vi "Automatic_IV_CV_with_XML_Global_Stop_V1.1.vi"() -> ()   [LabVIEW 2009]
uses:
  subVIs/CMSFPIX_LV80.llb/Keith 237 Operate/Standby.vi
  <vilib>/xml/Close Reference(Node).vi
  <vilib>/Utility/file.llb/Write To Spreadsheet File (string).vi
  <vilib>/Utility/file.llb/Write To Spreadsheet File (DBL).vi
  <vilib>/xml/NI_XML.lvlib
panel:
  in  "File Path":path=path "C:/Documents and Settings/PROBER/Desktop/Andrew_Test/VI Test Output"
  out "voltage \ncompliance level":dbl=1e-05
  out "Wafer Number":string
  out "Contact Check Result":string="Skipped"
  out "Site Number":i32
  out "File Name":string
  in  "Tab Control 2":enum32{"IV Check", "CV Check"}(tab)
  out "Boolean":bool caption="Voltage Breakdown"
  out "Boolean 2":bool caption="Leakage Current Check Total"
  out "Boolean 3":bool caption="Leakage Current Check Active"
  out "Boolean 4":bool caption="Leakage Current Check Guardring"
  out "Boolean 5":bool caption="150V Bias Check"
  out "Contact Check":bool
  out "Status":string
  out "Bias Polarity":dbl=1.0 format="%.2f"
  out "1/C^2":cluster{"Y":dbl[], "Y":dbl[]}[](graph)
  out "semaphore":T1
  out "voltage \ncompliance cutoff":dbl=1e-05
  in  "Tab Control":enum32{"Site Selection"}(tab)
  in  "Site 1":bool=TRUE
  in  "Site 2":bool=TRUE
  in  "Site 3":bool=TRUE
  in  "Site 4":bool=TRUE
  in  "Site 5":bool=TRUE
  in  "Site 6":bool=TRUE
  in  "Site 7":bool=TRUE
  in  "Site 8":bool=TRUE
  in  "Site 9":bool=TRUE
  in  "Site 10":bool=TRUE
  in  "Site 11":bool=TRUE
  in  "Site 12":bool=TRUE
  in  "Site 13":bool=TRUE
  in  "Site 14":bool=TRUE
  in  "Site 15":bool=TRUE
  in  "Site 16":bool=TRUE
  in  "Site 17":bool=TRUE
  in  "Site 18":bool=TRUE
  in  "Site 19":bool=TRUE
  in  "Site 20":bool=TRUE
  in  "Site 21":bool=TRUE
  in  "Site 22":bool=TRUE
  in  "Running Conditional":bool
  out "error out 7":T2
  in  "IV or CV":i32
  in  "Emergency Stop":bool
  out "error out 6":T2
  in  "Stop Loop":bool=TRUE
  in  "Total Site # CV":i32=12
  out "Secondary Parameter":u16(ring) items=["None", "Cs", "Cp", "Ls", "Lp", "Rs", "Rp", "DF", "Q", "Z", "Y", "Phase", "ESR", "Gp", "Xs", "Bp"]
  out "Auto Compliance":dbl=9.9e-05
  out "Compliance":dbl=1e-09
  out "Compliance":bool
  out "Total Current":dbl format="%#_6e"
  out "Secondary Parameter Graph":cluster{"Y":dbl[], "Y":dbl[]}[](graph) caption="DF"
  in  "Absolute?":bool
  out "Voltage Range":string
  out "Primary Parameter":u16(ring)=2 items=["AUTO", "Cs", "Cp", "Ls", "Lp", "Rs", "Rp", "DF", "Q", "Z", "Y", "Phase", "ESR", "Gp", "Xs", "Bp"]
  out "Time Delay mS":dbl=20.0
  out "Number of Averages":dbl=1.0
  out "Voltage Level":dbl=1.0
  out "Frequency":dbl=1000.0
  in  "Bias Loop":bool
  out "K237_Bias":dbl
  in  "Archive":T3(tab)=enum."Primary"
  out "Diode Total Current Archive":cluster{"Y":dbl[], "Y":dbl[]}[](graph) caption="Total Current"
  out "Diode GRD Archive":cluster{"Y":dbl[], "Y":dbl[]}[](graph)
  out "Diode ACTIVE Archive":cluster{"Y":dbl[], "Y":dbl[]}[](graph)
  out "Single Chip Total Current Archive":cluster{"Y":dbl[], "Y":dbl[]}[](graph) caption="Total Current"
  out "Single Chip GRD Archive":cluster{"Y":dbl[], "Y":dbl[]}[](graph)
  out "Single Chip ACTIVE Archive":cluster{"Y":dbl[], "Y":dbl[]}[](graph)
  out "2x8 Total Current Archive":cluster{"Y":dbl[], "Y":dbl[]}[](graph) caption="Total Current"
  out "2x8 GRD Archive":cluster{"Y":dbl[], "Y":dbl[]}[](graph)
  out "2x8 ACTIVE Archive":cluster{"Y":dbl[], "Y":dbl[]}[](graph)
  out "Slim-Edge ACTIVE Archive":cluster{"Y":dbl[], "Y":dbl[]}[](graph)
  out "Slim-Edge GRD Archive":cluster{"Y":dbl[], "Y":dbl[]}[](graph)
  out "Slim-Edge Total Current Archive":cluster{"Y":dbl[], "Y":dbl[]}[](graph) caption="Total Current"
  out "Single Chip Capacitance":cluster{"Y":dbl[], "Y":dbl[]}[](graph)
  out "2x8 Chip Capacitance":cluster{"Y":dbl[], "Y":dbl[]}[](graph)
  out "Diodes Capacitance":cluster{"Y":dbl[], "Y":dbl[]}[](graph)
  in  "Halt CV":bool
  in  "Halt IV":bool
  out "Running?":bool
  in  "Total Site # IV":i32=22
  out "Site # CV":dbl
  out "Site # IV":dbl
  out "error out":errorcluster
  in  "CV-V-Limit":i32=10
  out "Capacitance":cluster{"Y":dbl[], "Y":dbl[]}[](graph) caption="Cp"
  in  "CV-V-Steps":i32=1
  out "QuadTech Status":string
  out "Total Current":cluster{"Y":dbl[], "Y":dbl[]}[](graph)
  out "6485 GRD (GPIB 10)":cluster{"Y":dbl[], "Y":dbl[]}[](graph)
  out "6485 ACTIVE (GPIB 14)":cluster{"Y":dbl[], "Y":dbl[]}[](graph)
  out "error out 5":errorcluster
  out "error out 4":errorcluster
  in  "IV-V-Steps":i32=1
  in  "IV-V-Limit":i32=10
  in  "error in (no error)":errorcluster
  # "Note: The Total Site # indexes\nstarting at 0 and goes to n-1,\nso if there are a total of 3 sites\nthen Total Site # should be set\nto 3"
  # "Note 2: This code is setup for a specific\nwafer map. If a map with a different\nnumber of subsites and/or different layout\nis used the naming will be incorrect"
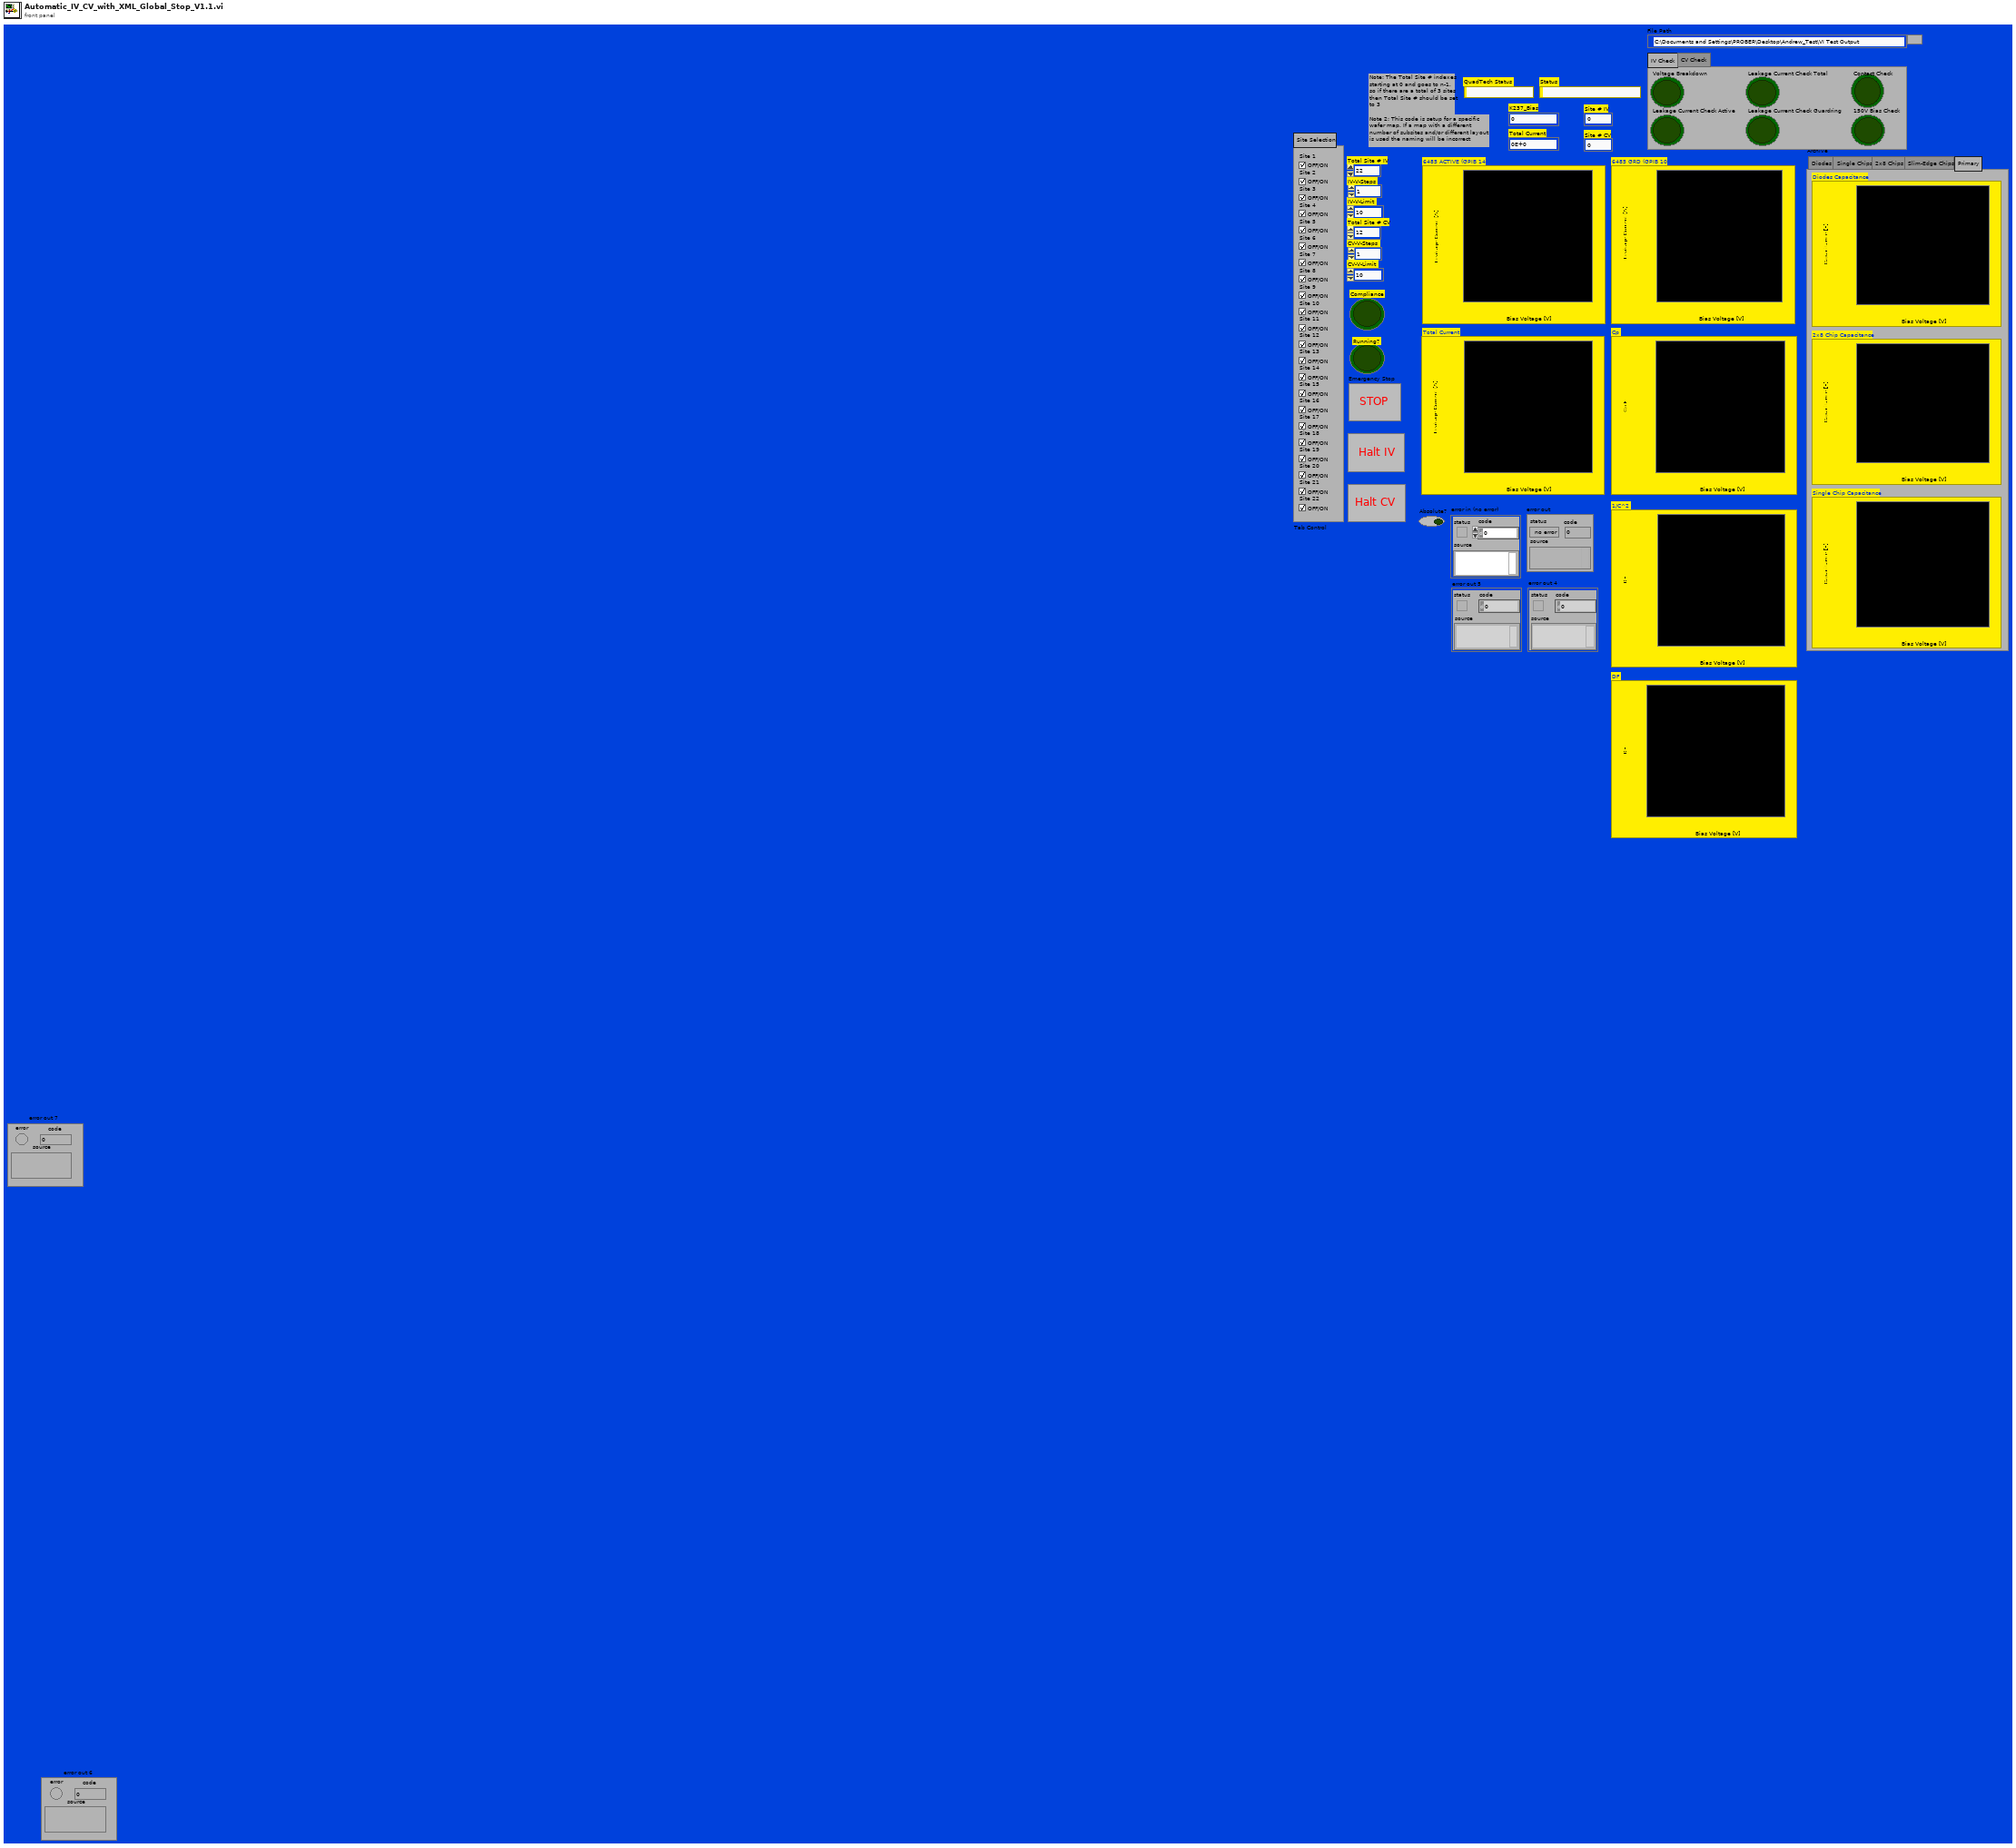
[diagram p1: front panel]
types:
  T1 = typedef "Semaphore RefNum" = refnum<k1>
  T2 = cluster{"error":bool, "code":i32, "source":string}
  T3 = enum32{"Diodes", "Single Chips", "2x8 Chips", "Slim-Edge Chips", "Primary"}
  T4 = cluster{"Name of Test":string, string, "Comment Description":string, "User":string}
  T5 = enum16{"open", "replace", "create", "open or create", "replace or create", "replace or create with confirmation"}
  T6 = cluster{cluster{"Y":dbl[], "Y":dbl[]}[], cluster{"Y":dbl[], "Y":dbl[]}[], cluster{"Y":dbl[], "Y":dbl[]}[], cluster{"Y":dbl[], "Y":dbl[]}[], cluster{"Y":dbl[], "Y":dbl[]}[], cluster{"Y":dbl[], "Y":dbl[]}[], cluster{"Y":dbl[], "Y":dbl[]}[], cluster{"Y":dbl[], "Y":dbl[]}[], cluster{"Y":dbl[], "Y":dbl[]}[], cluster{"Y":dbl[], "Y":dbl[]}[], cluster{"Y":dbl[], "Y":dbl[]}[], cluster{"Y":dbl[], "Y":dbl[]}[]}
  T7 = enum16{"Left Button", "Center Button", "Right Button", "Window Close"}
  T8 = cluster{"error":bool, "code":i8, "source":string}
  T9 = cluster{cluster{"Y":dbl[], "Y":dbl[]}[], cluster{"Y":dbl[], "Y":dbl[]}[], cluster{"Y":dbl[], "Y":dbl[]}[]}
  T10 = cluster{"Primary ":string, "Primary Value":string, "Primary Unit":string, "Secondary":string, "Secondary Value":string, "Secondary Unit":string}
  T11 = cluster{"XY Graph":cluster{"Y":dbl[], "Y":dbl[]}[], "XY Graph":cluster{"Y":dbl[], "Y":dbl[]}[], "XY Graph":cluster{"Y":dbl[], "Y":dbl[]}[]}
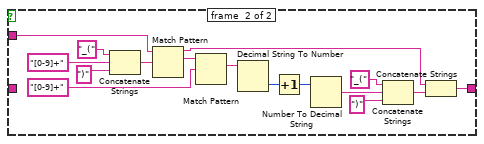
[diagram p2: hidden frame]
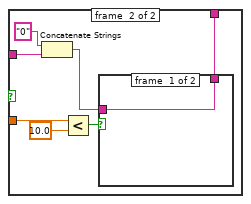
[diagram p4: hidden frame]
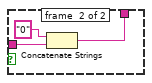
[diagram p5: hidden frame]
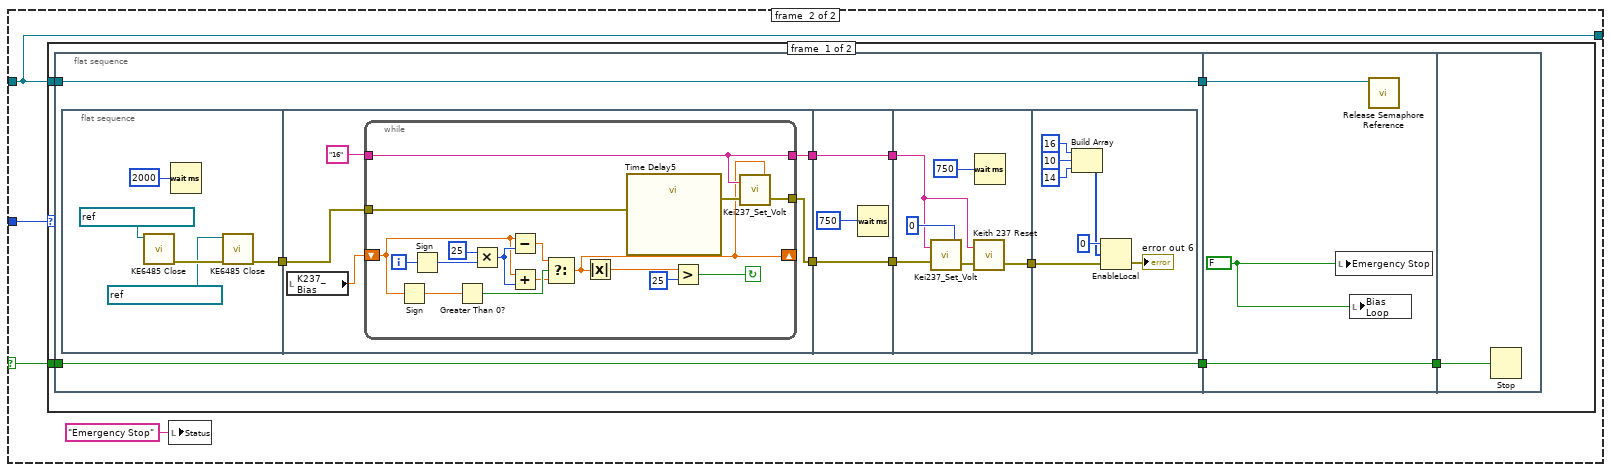
[diagram p7: hidden frame]
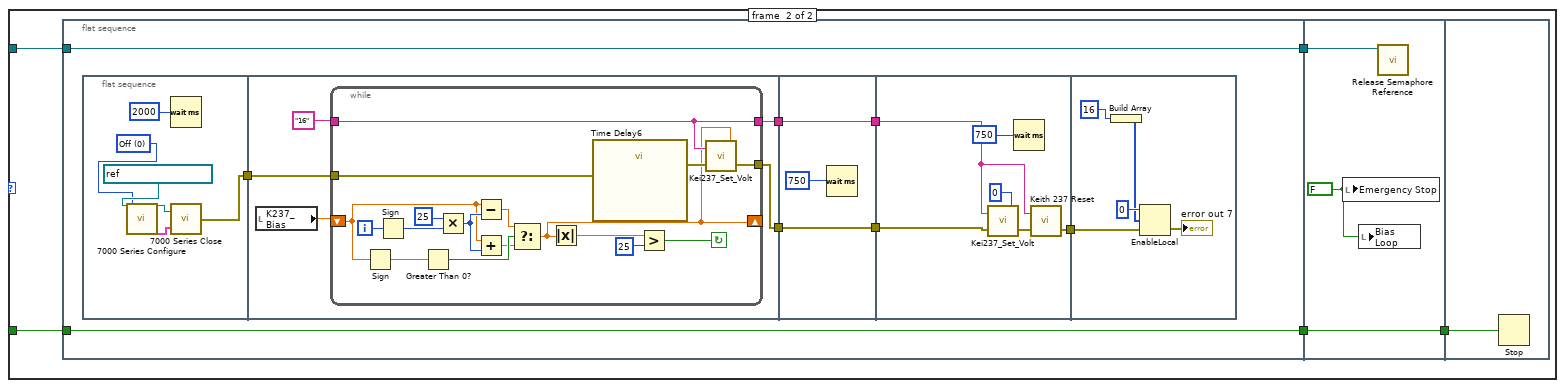
[diagram p8: hidden frame]
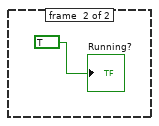
[diagram p9: hidden frame]
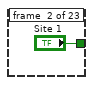
[diagram p10: hidden frame]
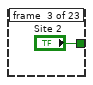
[diagram p11: hidden frame]
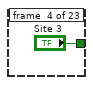
[diagram p12: hidden frame]
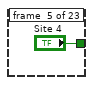
[diagram p13: hidden frame]
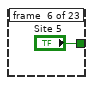
[diagram p14: hidden frame]
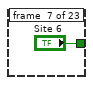
[diagram p15: hidden frame]
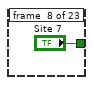
[diagram p16: hidden frame]
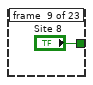
[diagram p17: hidden frame]
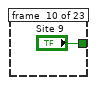
[diagram p18: hidden frame]
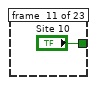
[diagram p19: hidden frame]
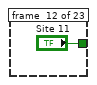
[diagram p20: hidden frame]
diagram:
  (unwired) path "" ("base path")
  # "Wafer Folder"
  # "Test Name Subfolder"
  # "XML Subfolder"
  # "Single Chip"
  # "2x8"
  # "Diode"
  # "Total"
  # "GRD"
  # "Active"
  # "Capacitance"
  # "Slim-Edge"
  # "2x8"
  # "Single Chip"
  # "Diodes"
  # "Change wiring to CV"
  # "DO CV MEASUREMENTS"
  # "Do CV measurements"
  # "Configure CV instuments"
  # "Do IV measurements"
  # "Configure IV instuments"
  # "DO IV MEASUREMENTS"
  n1 = invoke on="Diode ACTIVE Archive" class="XYGraph (strict)" method="Reinit To Default"() -> ()  [unwired: 3 in, 3 out]
  n2 = invoke on="Diode GRD Archive" class="XYGraph (strict)" method="Reinit To Default"() -> ()  [unwired: 3 in, 3 out]
  n3 = invoke on="Diode Total Current Archive" class="XYGraph (strict)" method="Reinit To Default"() -> ()  [unwired: 3 in, 3 out]
  n4 = invoke on="Diodes Capacitance" class="XYGraph (strict)" method="Reinit To Default"() -> ()  [unwired: 3 in, 3 out]
  n5 = invoke on="2x8 Chip Capacitance" class="XYGraph (strict)" method="Reinit To Default"() -> ()  [unwired: 3 in, 3 out]
  n6 = invoke on="Single Chip Capacitance" class="XYGraph (strict)" method="Reinit To Default"() -> ()  [unwired: 3 in, 3 out]
  n7 = invoke on="Single Chip ACTIVE Archive" class="XYGraph (strict)" method="Reinit To Default"() -> ()  [unwired: 3 in, 3 out]
  n8 = invoke on="Single Chip GRD Archive" class="XYGraph (strict)" method="Reinit To Default"() -> ()  [unwired: 3 in, 3 out]
  n9 = invoke on="Single Chip Total Current Archive" class="XYGraph (strict)" method="Reinit To Default"() -> ()  [unwired: 3 in, 3 out]
  n10 = invoke on="2x8 ACTIVE Archive" class="XYGraph (strict)" method="Reinit To Default"() -> ()  [unwired: 3 in, 3 out]
  n11 = invoke on="2x8 GRD Archive" class="XYGraph (strict)" method="Reinit To Default"() -> ()  [unwired: 3 in, 3 out]
  n12 = invoke on="2x8 Total Current Archive" class="XYGraph (strict)" method="Reinit To Default"() -> ()  [unwired: 3 in, 3 out]
  n13 = local write "K237_Bias"(0.0 ("K237_Bias")) -> ()
  n14 = invoke on="Slim-Edge ACTIVE Archive" class="XYGraph (strict)" method="Reinit To Default"() -> ()  [unwired: 3 in, 3 out]
  n15 = invoke on="Slim-Edge GRD Archive" class="XYGraph (strict)" method="Reinit To Default"() -> ()  [unwired: 3 in, 3 out]
  n16 = invoke on="Slim-Edge Total Current Archive" class="XYGraph (strict)" method="Reinit To Default"() -> ()  [unwired: 3 in, 3 out]
  n17 = call "Wafer ID"("error in (no error)"="error in (no error)") -> ("User"=w21:string, "Comment Description"=w22:string, "Name of Test"=w3:string, "Wafer ID #"=w15:dbl, "OK"=w63:bool, "error out"=w66:errorcluster)  [unwired: 13 in]
  n18 = Number To Decimal String(number=w15) -> (decimal integer string=w16:string)  [unwired: 1 in]
  n19 = Less?(x=w15, y=100.0) -> (x < y?=w18:bool)
  n20 = case shown="True" w18 {
    tunnel: w16 -> [w68 w75]
    tunnel: w15 -> [_ w72]
    tunnel: [w68 w69] -> w14
    frame #0 {
    }
    frame #1 {
      n21 = Concatenate Strings("0" ("string"), w75) -> (w70:string)
      n22 = Less?(x=w72, y=10.0) -> (x < y?=w73:bool)
      n23 = case shown="True" w73 {
        tunnel: w70 -> [w76 w79]
        tunnel: [w76 w77] -> w69
        frame #0 {
        }
        frame #1 {
          n24 = Concatenate Strings("0" ("string"), w79) -> (w77:string)
        }
      }
    }
  }
  "Wafer Number" <- w14
  n25 = Not(x=w63) -> (.not. x?=w62:bool)
  n26 = call <vilib>:"Obtain Semaphore Reference.vi"("size (1)"=1) -> ("semaphore"=w35:T1)  [unwired: 4 in, 2 out]
  "semaphore" <- w35
  n27 = Stop(stop? (T)=w62) -> ()
  n28 = Concatenate Strings("Wafer_" ("string"), w14) -> (w26:string)
  n29 = Build Path(base path="File Path", name or relative path=w26) -> (appended path=w25:path)
  n30 = Bundle("Name of Test"=w3, w14, "Comment Description"=w22, "User"=w21) -> (w13:T4)  [unwired: 1 in]
  n31 = flat-sequence {
    tunnel: w66 -> [w100]
    tunnel: [w98] -> w65
    tunnel: [w86] -> w59
    tunnel: [w88] -> w58
    tunnel: [w87] -> w57
    tunnel: [w91] -> w36
    tunnel: w35 -> [w91]
    tunnel: [w81] -> w19
    tunnel: w65 -> [w139]
    tunnel: w1 -> [w134]
    tunnel: w59 -> [w132]
    tunnel: w58 -> [w131]
    tunnel: w57 -> [w130]
    tunnel: [w129] -> w46
    tunnel: w36 -> [w122]
    tunnel: [w121] -> w29
    tunnel: w13 -> [w120]
    tunnel: w19 -> [w119]
    tunnel: w1 -> [w114]
    tunnel: w8 -> [w112]
    tunnel: w46 -> [w1232]
    tunnel: [w1232] -> w45
    tunnel: [w1230] -> w30
    tunnel: w29 -> [w1230]
    tunnel: [w1236] -> w47
    tunnel: w45 -> [w1237]
    tunnel: [w1234] -> w31
    tunnel: w30 -> [w1234]
    tunnel: w47 -> [w1246]
    tunnel: [w1246] -> w64
    tunnel: [w1242] -> w32
    tunnel: w31 -> [_]
    tunnel: w64 -> [w1255]
    tunnel: [w1254] -> w56
    tunnel: [w1253] -> w54
    tunnel: [w1252] -> w52
    tunnel: [w1250] -> w50
    tunnel: [w1249] -> w33
    tunnel: w32 -> [w1249]
    tunnel: w56 -> [w1289]
    tunnel: [w1289] -> w55
    tunnel: w54 -> [w1288]
    tunnel: [w1288] -> w53
    tunnel: w52 -> [w1287]
    tunnel: [w1287] -> w51
    tunnel: w50 -> [w1286]
    tunnel: ["Total Site # CV"] -> w38
    tunnel: [w1284] -> w34
    tunnel: w33 -> [w1284]
    tunnel: w55 -> [w1337]
    tunnel: w53 -> [w1336]
    tunnel: w51 -> [w1335]
    tunnel: w1 -> [w1327]
    tunnel: [FALSE ("Compliance")] -> w44
    tunnel: [TRUE ("Bias Loop")] -> w42
    tunnel: [w1325] -> w40
    tunnel: w38 -> [w1324]
    tunnel: w34 -> [w1323]
    tunnel: w13 -> [w1321]
    tunnel: w8 -> [w1320]
    tunnel: w44 -> [w1897]
    tunnel: [w1897] -> w43
    tunnel: w42 -> [w1900]
    tunnel: [w1900] -> w41
    tunnel: w40 -> [w1899]
    tunnel: [w1899] -> w39
    tunnel: [w1908] -> w48
    tunnel: [w1909] -> w49
    tunnel: w43 -> [w1909]
    tunnel: w41 -> [w1908]
    tunnel: w39 -> [w1903]
    frame #0 {
      w81 = 0 ("Numeric")
      w92 = FALSE
      w101 = u16 5 items=["auto / auto", "1 nA / 1.1 V", "10 nA / 11 V", "100 nA / 110 V", "0.001 mA / 1100 V", "0.01 mA / 1100 V", "0.1 mA / 1100 V", "1 mA / 1100 V", "10 mA / 1100 V", "100 mA / 1100 V"] ("source range\nI source / V source (auto:0)")
      w104 = u16 0 items=["voltage/current", "current/voltage"] ("source/measure (V/I:0)")
      w105 = u16 5 items=["auto / auto", "1 nA / 1.1 V", "10 nA / 11 V", "100 nA / 110 V", "0.001 mA / 1100 V", "0.01 mA / 1100 V", "0.1 mA / 1100 V", "1 mA / 1100 V", "10 mA / 1100 V", "100 mA / 1100 V"] ("compliance/\nmeasurement range (auto:0)")
      w103 = 3e-05 ("voltage \ncompliance level")
      w108 = u16 0 items=["DC", "sweep"] ("function (DC:0)")
      w98 = "16"  # GPIB
      # "Change Bias Polarity\n+1 Chuck Bias\n-1  Pad bias"
      # "Keithley 237 as sourcemeter\nKeithley 6485 as picoammeters"
      n32 = call "Keith 237 Reset.vi"("GPIB address"=w98, "error in"=w100) -> ("error out"=w99:T2)
      n33 = call "Keith 237 Basic Config.vi"("GPIB address"=w98, "source/measure (V/I:0)"=w104, "function (DC:0)"=w108, "source range\nI source / V source (auto:0)"=w101, "source level"=0.0, "error in"=w99, "1100 V range (disabled:F)"=TRUE, "current \ncompliance level"=w103, "compliance/\nmeasurement range (auto:0)"=w105) -> ("error out"=w110:T2)  [unwired: 7 in, 3 out]
      n34 = local write "IV or CV"(w81) -> ()
      n35 = call "Keith 237 Operate/Standby.vi"("source"=FALSE, "error in"=w110, "GPIB address"=w98) -> ("error out"=w109:T2)
      n36 = Multiply(x=w103, y=0.98 ("voltage \ncompliance level")) -> (x*y=→"voltage \ncompliance cutoff":dbl)
      n37 = call "Keith 237 Send Trigger.vi"("GPIB address"=w98, "error in"=w109) -> ("error out"=w96:T2)
      n38 = call "KE6485 Initialize.vi"("error in (no error)"=w96, "resource name"=refnum<k15> "GPIB0::10::INSTR" ("instrument handle")) -> ("error out"=w90:errorcluster, "instrument handle out"=w93:refnum<k15>)  [unwired: 8 in]
      n39 = property class="KE6485"(reference=w93, error in=w90, "System Settings:Zero Check Enabled"=w92) -> (reference out=w86:refnum<k15>, error out=w85:errorcluster)
      n40 = call "KE6485 Initialize.vi"("error in (no error)"=w85, "resource name"=refnum<k15> "GPIB0::14::INSTR" ("instrument handle")) -> ("error out"=w89:errorcluster, "instrument handle out"=w94:refnum<k15>)  [unwired: 8 in]
      n41 = property class="KE6485"(reference=w94, error in=w89, "System Settings:Zero Check Enabled"=w92) -> (reference out=w88:refnum<k15>, error out=w87:errorcluster)
      "Bias Polarity" <- 1.0
      "Status" <- "Setting IV Scan Parameters" ("Status")
      "voltage \ncompliance level" <- w103
    }
    frame #1 {
      w123 = cluster{"Y":dbl[], "Y":dbl[]}[] []
      # "10"
      # "14"
      n42 = Build Path(base path=w114, name or relative path="Contact_Check.csv") -> (appended path=w118:path)
      n43 = Open/Create/Replace File(file path (use dialog)=w118, operation (0:open)=T5."replace or create", access (0:read/write)=enum16{"read/write", "read-only", "write-only"}."read/write") -> (refnum out=w117:refnum<file>)  [unwired: 1 in, 4 out]
      n44 = Refnum to Path(1:w117) -> (0:w113:path)
      n45 = for {
        N: "Total Site # IV" -> [_]
        tunnel: w139 -> [w233]
        tunnel: "IV-V-Limit" -> [w235]
        tunnel: "IV-V-Steps" -> [w236]
        tunnel: [w232] -> w137
        shift-right: [w231] -> w125
        shift-left: w130 -> [w234]
        shift-right: [w226] -> _
        shift-left: w123 -> [w197]
        shift-right: [w225] -> _
        shift-left: w123 -> [w196]
        shift-right: [w224] -> _
        shift-left: w123 -> [w195]
        shift-right: [w223] -> _
        shift-left: w123 -> [w194]
        shift-right: [w222] -> _
        shift-left: w123 -> [w189]
        shift-right: [w221] -> _
        shift-left: w123 -> [w193]
        shift-right: [w220] -> _
        shift-left: w123 -> [w192]
        shift-right: [w200] -> _
        shift-left: w123 -> [w191]
        shift-right: [w219] -> _
        shift-left: w123 -> [w190]
        tunnel: w134 -> [w202]
        tunnel: "Absolute?" -> [w201]
        tunnel: w132 -> [w199]
        tunnel: w131 -> [w198]
        shift-right: [w184] -> _
        shift-left: w123 -> [w187]
        shift-right: [w183] -> _
        shift-left: w123 -> [w186]
        shift-right: [w182] -> _
        shift-left: w123 -> [w185]
        tunnel: w122 -> [w181]
        tunnel: [w180] -> w121
        tunnel: w120 -> [w165]
        tunnel: w119 -> [w167]
        tunnel: w113 -> [w143]
        tunnel: w112 -> [w141]
        i -> [w166]
        (unwired) TRUE
        # "User Input Array\nElement 0: Comment Description (XML_Header)\nElement 1: Serial Number\nElement 2: Kind of Part\nElement 3: User\nElement 4: Extension Table Name\nElement 5: Comment Description (XML_Data_Set)\nElement 6: Name (XML_Header)\nElement 7: Run Name (XML_Header)"
        # "XML Data Tags for IV scan"
        n46 = Increment(x=w166) -> (x+1=→"Site # IV":i32)
        n47 = Bundle(w197, w196, w195, w194, w193, w192, w191, w190, w189, w187, w186, w185) -> (w188:T6)  [unwired: 1 in]
        n48 = flat-sequence {
          tunnel: [w247] -> w151
          tunnel: w234 -> [w247]
          tunnel: [w246] -> w153
          tunnel: w233 -> [w246]
          tunnel: w166 -> [w238]
          tunnel: [w245] -> w155
          tunnel: w199 -> [w245]
          tunnel: [w244] -> w157
          tunnel: w198 -> [w244]
          tunnel: w181 -> [w243]
          tunnel: [w243] -> w159
          tunnel: [w237] -> w149
          tunnel: [w239] -> w148
          tunnel: [w241] -> w146
          tunnel: [w238] -> w142
          tunnel: w159 -> [w289]
          tunnel: [w288] -> w158
          tunnel: w157 -> [w287]
          tunnel: [w286] -> w156
          tunnel: w155 -> [w285]
          tunnel: [w284] -> w154
          tunnel: w153 -> [w282]
          tunnel: [w281] -> w152
          tunnel: w151 -> [w283]
          tunnel: [w280] -> w150
          tunnel: w149 -> [w272]
          tunnel: w148 -> [w276]
          tunnel: [w276] -> w147
          tunnel: w146 -> [w277]
          tunnel: [w277] -> w145
          tunnel: [w279] -> w144
          tunnel: w142 -> [w273]
          tunnel: w236 -> [w557]
          tunnel: w235 -> [w556]
          tunnel: [w553] -> w208
          tunnel: [w552] -> w207
          tunnel: [w545] -> w206
          tunnel: [w551] -> w205
          tunnel: [w550] -> w204
          tunnel: w218 -> [w549]
          tunnel: w169 -> [w547]
          tunnel: w209 -> [w546]
          tunnel: [w541] -> w203
          tunnel: w201 -> [w544]
          tunnel: [w539] -> w180
          tunnel: w158 -> [w540]
          tunnel: w156 -> [w542]
          tunnel: w154 -> [w543]
          tunnel: w152 -> [w554]
          tunnel: w150 -> [w555]
          tunnel: w147 -> [w534]
          tunnel: w145 -> [w532]
          tunnel: w160 -> [w538]
          tunnel: w140 -> [w537]
          tunnel: w161 -> [w536]
          tunnel: w144 -> [w535]
          tunnel: w140 -> [w530]
          tunnel: w208 -> [w931]
          tunnel: [w930] -> w179
          tunnel: w207 -> [w927]
          tunnel: [w929] -> w177
          tunnel: w206 -> [w934]
          tunnel: [w934] -> w175
          tunnel: w205 -> [w933]
          tunnel: [w933] -> w173
          tunnel: w204 -> [w932]
          tunnel: [w932] -> w171
          tunnel: w203 -> [w928]
          tunnel: w179 -> [w963]
          tunnel: [w963] -> w178
          tunnel: w177 -> [w962]
          tunnel: [w962] -> w176
          tunnel: w175 -> [w961]
          tunnel: [w961] -> w174
          tunnel: w173 -> [w960]
          tunnel: [w960] -> w172
          tunnel: w171 -> [w959]
          tunnel: [w959] -> w170
          tunnel: [w984] -> w231
          tunnel: [w986] -> w232
          tunnel: w178 -> [w986]
          tunnel: w176 -> [w1023]
          tunnel: w166 -> [w1018]
          tunnel: w174 -> [w1017]
          tunnel: w172 -> [w1016]
          tunnel: w170 -> [w1015]
          tunnel: [w1014] -> w226
          tunnel: [w1013] -> w225
          tunnel: [w1012] -> w224
          tunnel: [w1011] -> w223
          tunnel: [w1010] -> w222
          tunnel: [w1009] -> w221
          tunnel: [w1008] -> w220
          tunnel: [w1007] -> w200
          tunnel: [w1006] -> w219
          tunnel: w188 -> [w1004]
          tunnel: [w990] -> w184
          tunnel: [w989] -> w183
          tunnel: [w988] -> w182
          tunnel: w143 -> [w968]
          frame #0 {
            n49 = Increment(x=w238) -> (x+1=w242:i32)
            n50 = case shown="1" w242 {
              tunnel: [TRUE "Site 1" "Site 2" "Site 3" "Site 4" "Site 5" "Site 6" "Site 7" "Site 8" "Site 9" "Site 10" "Site 11" "Site 12" "Site 13" "Site 14" "Site 15" "Site 16" "Site 17" "Site 18" "Site 19" "Site 20" "Site 21" "Site 22"] -> w239
              frame #0 {
              }
              frame #1 {
              }
              frame #2 {
              }
              frame #3 {
              }
              frame #4 {
              }
              frame #5 {
              }
              frame #6 {
              }
              frame #7 {
              }
              frame #8 {
              }
              frame #9 {
              }
              frame #10 {
              }
              frame #11 {
              }
              frame #12 {
              }
              frame #13 {
              }
              frame #14 {
              }
              frame #15 {
              }
              frame #16 {
              }
              frame #17 {
              }
              frame #18 {
              }
              frame #19 {
              }
              frame #20 {
              }
              frame #21 {
              }
              frame #22 {
              }
            }
            n51 = Wait (ms)(milliseconds to wait=u32 250) -> ()  [unwired: 1 out]
            n52 = Increment(x=w238) -> (x+1=w237:i32)
            n53 = call "Skip Current Subsite"("Enable"=w239) -> ("Skip Subsite"=w241:bool)  [unwired: 17 in, 1 out]
          }
          frame #1 {
            w271 = FALSE ("Visible")
            n54 = local write "Contact Check"(w271) -> ()
            n55 = local write "Boolean 2"(w271) -> ()
            n56 = local write "Boolean 3"(w271) -> ()
            n57 = local write "Boolean 4"(w271) -> ()
            n58 = local write "Boolean 5"(w271) -> ()
            n59 = local write "Boolean"(w271) -> ()
            n60 = Not(x=w276) -> (.not. x?=w275:bool)
            n61 = property on="Tab Control 2" class="TabCtl (strict)"("Visible"=TRUE) -> ()  [unwired: 2 in, 2 out]
            n62 = Compound Arithmetic op=OR(w275, w277) -> (w278:bool)
            n63 = case shown="False" w278 {
              tunnel: w289 -> [w302 w525]
              tunnel: [w301 w525] -> w288
              tunnel: w287 -> [w300 w526]
              tunnel: [w299 w526] -> w286
              tunnel: w285 -> [w298 w527]
              tunnel: [w297 w527] -> w284
              tunnel: w272 -> [w296 w523]
              tunnel: w283 -> [w295 w528]
              tunnel: w282 -> [w294 w529]
              tunnel: [w293 w529] -> w281
              tunnel: [w292 w528] -> w280
              tunnel: [w291 TRUE] -> w279
              tunnel: w273 -> [w290 _]
              frame #0 {
                n64 = flat-sequence {
                  tunnel: w302 -> [w318]
                  tunnel: w300 -> [w317]
                  tunnel: w298 -> [w316]
                  tunnel: w296 -> [w313]
                  tunnel: [w318] -> w307
                  tunnel: [w317] -> w306
                  tunnel: [w316] -> w305
                  tunnel: [w312] -> w304
                  tunnel: w294 -> [w312]
                  tunnel: [w311] -> w303
                  tunnel: w295 -> [w311]
                  tunnel: w290 -> [w308]
                  tunnel: [w326] -> w297
                  tunnel: [w325] -> w299
                  tunnel: [w323] -> w301
                  tunnel: w307 -> [w324]
                  tunnel: w306 -> [w332]
                  tunnel: w305 -> [w331]
                  tunnel: w304 -> [w330]
                  tunnel: w303 -> [w329]
                  tunnel: [w328] -> w293
                  tunnel: [w327] -> w292
                  tunnel: [w322] -> w291
                  frame #0 {
                    # "Go to N subsite"
                    n65 = Number To Decimal String(number=w308) -> (decimal integer string=w315:string)  [unwired: 1 in]
                    n66 = local write "Contact Check Result"("Not Skipped" ("Contact Check Result")) -> ()
                    n67 = Wait (ms)(milliseconds to wait=u32 1500) -> ()  [unwired: 1 out]
                    n68 = call "-mov-prob-abs-subs.vi"("Subsite #"=w315) -> ()  [unwired: 5 in]
                    n69 = local write "Status"("Moving to Subsite" ("Status")) -> ()
                    "Site Number" <- w313
                  }
                  frame #1 {
                    n70 = local read "Bias Polarity"() -> (w320:dbl)
                    n71 = Wait (ms)(milliseconds to wait=u32 500) -> ()  [unwired: 1 out]
                    n72 = Multiply(x=w320, y=3.0) -> (x*y=w319:dbl)
                    n73 = local write "Status"("IV Contact Check" ("Status")) -> ()
                    n74 = while {
                      tunnel: w332 -> [w347]
                      tunnel: w331 -> [w346]
                      tunnel: w330 -> [w345]
                      tunnel: w329 -> [w344]
                      tunnel: [w343] -> w328
                      tunnel: [w342] -> w327
                      tunnel: [w341] -> w326
                      tunnel: [w340] -> w325
                      tunnel: w324 -> [w339]
                      tunnel: [w338] -> w323
                      tunnel: [w337] -> w322
                      tunnel: w319 -> [w336]
                      stop <- w335 stop-if-true
                      # "Contact Check"
                      n75 = flat-sequence {
                        tunnel: w347 -> [w405]
                        tunnel: w346 -> [w406]
                        tunnel: w344 -> [w407]
                        tunnel: [w407] -> w400
                        tunnel: [w406] -> w399
                        tunnel: [w405] -> w398
                        tunnel: [w404] -> w397
                        tunnel: w339 -> [w403]
                        tunnel: w345 -> [w402]
                        tunnel: [w402] -> w396
                        tunnel: [w401] -> w395
                        tunnel: w336 -> [w401]
                        tunnel: w400 -> [w413]
                        tunnel: [w412] -> w394
                        tunnel: w399 -> [w416]
                        tunnel: [w416] -> w393
                        tunnel: w398 -> [w415]
                        tunnel: [w415] -> w392
                        tunnel: w397 -> [w414]
                        tunnel: [w414] -> w391
                        tunnel: w396 -> [w410]
                        tunnel: [w410] -> w390
                        tunnel: w395 -> [w409]
                        tunnel: [w408] -> w389
                        tunnel: [w423] -> w388
                        tunnel: [w421] -> w387
                        tunnel: [w420] -> w386
                        tunnel: w394 -> [w422]
                        tunnel: w393 -> [w421]
                        tunnel: w392 -> [w420]
                        tunnel: [w419] -> w385
                        tunnel: w391 -> [w419]
                        tunnel: [w418] -> w384
                        tunnel: w390 -> [w418]
                        tunnel: w389 -> [w417]
                        tunnel: w388 -> [w429]
                        tunnel: w387 -> [w428]
                        tunnel: w386 -> [w427]
                        tunnel: [w429] -> w383
                        tunnel: [w428] -> w382
                        tunnel: [w427] -> w381
                        tunnel: w385 -> [w426]
                        tunnel: [w425] -> w380
                        tunnel: [w424] -> w379
                        tunnel: w384 -> [w424]
                        tunnel: w383 -> [w432]
                        tunnel: w382 -> [w435]
                        tunnel: w381 -> [w434]
                        tunnel: [w431] -> w378
                        tunnel: [w435] -> w377
                        tunnel: [w434] -> w376
                        tunnel: [w433] -> w375
                        tunnel: w380 -> [w433]
                        tunnel: [w430] -> w374
                        tunnel: w379 -> [w430]
                        tunnel: w378 -> [w441]
                        tunnel: w377 -> [w440]
                        tunnel: w376 -> [w439]
                        tunnel: [w441] -> w373
                        tunnel: [w440] -> w372
                        tunnel: [w439] -> w371
                        tunnel: w375 -> [w438]
                        tunnel: [w437] -> w370
                        tunnel: [w436] -> w369
                        tunnel: w374 -> [w436]
                        tunnel: w373 -> [w451]
                        tunnel: w372 -> [w446]
                        tunnel: w371 -> [w445]
                        tunnel: [w448] -> w368
                        tunnel: [w447] -> w367
                        tunnel: w370 -> [w447]
                        tunnel: w369 -> [w444]
                        tunnel: [w446] -> w366
                        tunnel: [w445] -> w365
                        tunnel: [w444] -> w364
                        tunnel: [w443] -> w363
                        tunnel: [w442] -> w362
                        tunnel: w368 -> [w458]
                        tunnel: [w461] -> w361
                        tunnel: w367 -> [w464]
                        tunnel: [w464] -> w360
                        tunnel: w366 -> [w463]
                        tunnel: [w463] -> w359
                        tunnel: w365 -> [w462]
                        tunnel: [w462] -> w358
                        tunnel: w364 -> [w457]
                        tunnel: [w457] -> w357
                        tunnel: w363 -> [w455]
                        tunnel: [w454] -> w356
                        tunnel: w362 -> [w453]
                        tunnel: [w452] -> w355
                        tunnel: w361 -> [w472]
                        tunnel: w360 -> [w471]
                        tunnel: w359 -> [w469]
                        tunnel: w358 -> [w468]
                        tunnel: w357 -> [w467]
                        tunnel: [w472] -> w354
                        tunnel: [w470] -> w353
                        tunnel: [w469] -> w352
                        tunnel: [w468] -> w351
                        tunnel: [w467] -> w350
                        tunnel: w356 -> [w466]
                        tunnel: [w466] -> w349
                        tunnel: w355 -> [w465]
                        tunnel: [w465] -> w348
                        tunnel: [w482] -> w343
                        tunnel: [w483] -> w340
                        tunnel: [w484] -> w341
                        tunnel: [w485] -> w338
                        tunnel: [w486] -> w342
                        tunnel: w354 -> [w486]
                        tunnel: w353 -> [w485]
                        tunnel: w352 -> [w484]
                        tunnel: w351 -> [w483]
                        tunnel: w350 -> [w482]
                        tunnel: w349 -> [w478]
                        tunnel: w348 -> [w477]
                        tunnel: [w476] -> w337
                        tunnel: [w473] -> w335
                        frame #0 {
                          n76 = call <vilib>:"Acquire Semaphore.vi"("semaphore"=w403) -> ("semaphore out"=w404:T1)  [unwired: 4 in, 2 out]
                        }
                        frame #1 {
                          n77 = call "Keith 237 Operate/Standby.vi"("source"=TRUE, "error in"=w413, "GPIB address"=w410) -> ("error out"=w412:T2)
                          n78 = Negate(x=w409) -> (-x=w408:dbl)
                        }
                        frame #2 {
                          n79 = call "Kei237_Set_Volt.vi"("Voltage"=w417, "error in"=w422, "GPIB"=w418) -> ("error out"=w423:errorcluster)
                          n80 = local write "K237_Bias"(w417) -> ()
                        }
                        frame #3 {
                          n81 = call <vilib>:"Release Semaphore.vi"("semaphore"=w426) -> ("semaphore out"=w425:T1)  [unwired: 5 in, 1 out]
                        }
                        frame #4 {
                          n82 = call "Time Delay7"("error in (no error)"=w432) -> ("error out"=w431:errorcluster)  [unwired: 10 in]
                        }
                        frame #5 {
                          n83 = call <vilib>:"Acquire Semaphore.vi"("semaphore"=w438) -> ("semaphore out"=w437:T1)  [unwired: 4 in, 2 out]
                        }
                        frame #6 {
                          # "14"
                          # "10"
                          n84 = call "K237-read-current-2.vi"("error in"=w451, "GPIB"=w444) -> ("error out"=w450:T2)  [unwired: 1 out]
                          n85 = call "KE6485 Read.vi"("error in (no error)"=w450, "instrument handle"=w446) -> ("error out"=w449:errorcluster, "reading"=w443:dbl)  [unwired: 7 in, 1 out]
                          n86 = call "KE6485 Read.vi"("error in (no error)"=w449, "instrument handle"=w445) -> ("error out"=w448:errorcluster, "reading"=w442:dbl)  [unwired: 7 in, 1 out]
                        }
                        frame #7 {
                          n87 = call "Kei237_Set_Volt.vi"("Voltage"=0.0, "error in"=w458, "GPIB"=w457) -> ("error out"=w459:errorcluster)
                          n88 = Absolute Value(x=w453) -> (abs(x)=w452:dbl)
                          n89 = Absolute Value(x=w455) -> (abs(x)=w454:dbl)
                          n90 = call "Keith 237 Operate/Standby.vi"("source"=FALSE, "error in"=w459, "GPIB address"=w457) -> ("error out"=w461:T2)
                        }
                        frame #8 {
                          n91 = call <vilib>:"Release Semaphore.vi"("semaphore"=w471) -> ("semaphore out"=w470:T1)  [unwired: 5 in, 1 out]
                        }
                        frame #9 {
                          w479 = 1e-06
                          n92 = Greater?(x=w478, y=w479) -> (0:w481:bool)
                          n93 = Greater?(x=w477, y=w479) -> (0:w480:bool)
                          n94 = And(x=w481, y=w480) -> (x .and. y?=w475:bool)
                          "Contact Check" <- w475
                          n95 = local read "Site Number"() -> (w474:i32)
                          n96 = case shown="False" w475 {
                            selector: w475 -> [_ w520]
                            tunnel: [w509 FALSE] -> w476
                            tunnel: [w509 w520] -> w473
                            frame #0 {
                              n97 = call <vilib>:"Three Button Dialog.vi"("Window Title (\"\")"="Contact Check Failed" ("Window Title (\"\")"), "Right Button Text (\"Cancel\")"="Retry" ("Right Button Text (\"Cancel\")"), "Center Button Text (\"No\")"="Global Stop" ("Center Button Text (\"No\")"), "Left Button Text (\"Yes\")"="Skip Subsite" ("Left Button Text (\"Yes\")"), "message"="Warning: If the light needs to be turned on make sure the K237 is in Standby") -> ("Which Button?"=w511:T7)  [unwired: 6 in]
                              n98 = case shown="\"Right Button\"" w511 {
                                tunnel: [TRUE w518 FALSE] -> w509
                                frame #0 {
                                }
                                frame #1 {
                                w518 = TRUE
                                n99 = local write "Emergency Stop"(w518) -> ()
                                n100 = Wait (ms)(milliseconds to wait=u32 3000) -> ()  [unwired: 1 out]
                                }
                                frame #2 {
                                }
                              }
                            }
                            frame #1 {
                            }
                          }
                          n101 = case shown="1" w474 {
                            tunnel: w475 -> [_ w487 w488 w489 w490 w491 w492 w493 w494 w495 w496 w497 w498 w499 w500 w501 w502 w503 w504 w505 w506 w507 w508]
                            frame #0 {
                              (unwired) TRUE
                            }
                            frame #1 {
                              n102 = local write "Site 1"(w487) -> ()
                            }
                            frame #2 {
                              n103 = local write "Site 2"(w488) -> ()
                            }
                            frame #3 {
                              n104 = local write "Site 3"(w489) -> ()
                            }
                            frame #4 {
                              n105 = local write "Site 4"(w490) -> ()
                            }
                            frame #5 {
                              n106 = local write "Site 5"(w491) -> ()
                            }
                            frame #6 {
                              n107 = local write "Site 6"(w492) -> ()
                            }
                            frame #7 {
                              n108 = local write "Site 7"(w493) -> ()
                            }
                            frame #8 {
                              n109 = local write "Site 8"(w494) -> ()
                            }
                            frame #9 {
                              n110 = local write "Site 9"(w495) -> ()
                            }
                            frame #10 {
                              n111 = local write "Site 10"(w496) -> ()
                            }
                            frame #11 {
                              n112 = local write "Site 11"(w497) -> ()
                            }
                            frame #12 {
                              n113 = local write "Site 12"(w498) -> ()
                            }
                            frame #13 {
                              n114 = local write "Site 13"(w499) -> ()
                            }
                            frame #14 {
                              n115 = local write "Site 14"(w500) -> ()
                            }
                            frame #15 {
                              n116 = local write "Site 15"(w501) -> ()
                            }
                            frame #16 {
                              n117 = local write "Site 16"(w502) -> ()
                            }
                            frame #17 {
                              n118 = local write "Site 17"(w503) -> ()
                            }
                            frame #18 {
                              n119 = local write "Site 18"(w504) -> ()
                            }
                            frame #19 {
                              n120 = local write "Site 19"(w505) -> ()
                            }
                            frame #20 {
                              n121 = local write "Site 20"(w506) -> ()
                            }
                            frame #21 {
                              n122 = local write "Site 21"(w507) -> ()
                            }
                            frame #22 {
                              n123 = local write "Site 22"(w508) -> ()
                            }
                          }
                        }
                      }
                    }
                  }
                }
              }
              frame #1 {
                n124 = local write "Site Number"(w523) -> ()
                "Contact Check Result" <- "Skipped"
              }
            }
          }
          frame #2 {
            n125 = Not(x=w534) -> (.not. x?=w533:bool)
            n126 = Compound Arithmetic op=OR(w535, w533, w532) -> (w531:bool)
            n127 = case shown="False" w531 {
              tunnel: w557 -> [w655 _]
              tunnel: w556 -> [w654 _]
              tunnel: w555 -> [w653 w924]
              tunnel: w554 -> [w652 w925]
              tunnel: [w651 w925] -> w553
              tunnel: [w650 w924] -> w552
              tunnel: [w649 w922] -> w551
              tunnel: [w648 w922] -> w550
              tunnel: w549 -> [w647 w921]
              tunnel: [w646 w921] -> w548
              tunnel: w547 -> [w645 _]
              tunnel: w546 -> [w578 _]
              tunnel: [w644 w922] -> w545
              tunnel: w544 -> [w643 _]
              tunnel: w543 -> [w642 _]
              tunnel: w542 -> [w641 _]
              tunnel: [w640 0] -> w541
              tunnel: w540 -> [w639 w920]
              tunnel: [w638 w920] -> w539
              tunnel: w538 -> [w624 _]
              tunnel: w537 -> [w623 _]
              tunnel: w536 -> [w621 _]
              tunnel: w530 -> [w577 _]
              frame #0 {
                (unwired) FALSE
                # "Read \nCurrent"
                # "Set Voltage"
                n128 = flat-sequence {
                  tunnel: [w665] -> w636
                  tunnel: [w664] -> w635
                  tunnel: [w669] -> w634
                  tunnel: [w668] -> w633
                  tunnel: [w667] -> w632
                  tunnel: [w661] -> w631
                  tunnel: w653 -> [w666]
                  tunnel: w652 -> [w664]
                  tunnel: w642 -> [w669]
                  tunnel: w641 -> [w668]
                  tunnel: w639 -> [w667]
                  tunnel: w655 -> [w693]
                  tunnel: w654 -> [w692]
                  tunnel: w622 -> [w688]
                  tunnel: w647 -> [w685]
                  tunnel: w645 -> [w683]
                  tunnel: w578 -> [w682]
                  tunnel: w643 -> [w680]
                  tunnel: w636 -> [w691]
                  tunnel: w635 -> [w674]
                  tunnel: w634 -> [w679]
                  tunnel: w633 -> [w678]
                  tunnel: w632 -> [w676]
                  tunnel: w631 -> [w672]
                  tunnel: [w690] -> w576
                  tunnel: [w689] -> w574
                  tunnel: [w687] -> w572
                  tunnel: [w686] -> w570
                  tunnel: [w684] -> w568
                  tunnel: [w681] -> w566
                  tunnel: [w677] -> w564
                  tunnel: [w675] -> w562
                  tunnel: [w671] -> w560
                  tunnel: [w670] -> w558
                  tunnel: w576 -> [w886]
                  tunnel: [w886] -> w575
                  tunnel: w574 -> [w885]
                  tunnel: [w885] -> w573
                  tunnel: w572 -> [w884]
                  tunnel: [w884] -> w571
                  tunnel: w570 -> [w883]
                  tunnel: [w883] -> w569
                  tunnel: w568 -> [w882]
                  tunnel: [w882] -> w567
                  tunnel: w566 -> [w881]
                  tunnel: [w881] -> w565
                  tunnel: w564 -> [w880]
                  tunnel: [w880] -> w563
                  tunnel: w562 -> [w879]
                  tunnel: [w879] -> w561
                  tunnel: w560 -> [w878]
                  tunnel: [w878] -> w559
                  tunnel: w558 -> [w877]
                  tunnel: [w911] -> w638
                  tunnel: [w912] -> w640
                  tunnel: [w913] -> w644
                  tunnel: [w914] -> w646
                  tunnel: [w915] -> w648
                  tunnel: [w916] -> w649
                  tunnel: [w917] -> w650
                  tunnel: [w918] -> w651
                  tunnel: w575 -> [w918]
                  tunnel: w573 -> [w917]
                  tunnel: w571 -> [w916]
                  tunnel: w569 -> [w915]
                  tunnel: w567 -> [w914]
                  tunnel: w565 -> [w913]
                  tunnel: w563 -> [w912]
                  tunnel: w561 -> [w911]
                  tunnel: w559 -> [w910]
                  tunnel: w621 -> [w909]
                  tunnel: [w889] -> w614
                  tunnel: [w887] -> w580
                  frame #0 {
                    n129 = local read "Bias Polarity"() -> (w661:dbl)
                    n130 = call "Keith 237 Operate/Standby.vi"("source"=TRUE, "error in"=w666, "GPIB address"=w664) -> ("error out"=w665:T2)
                    n131 = Wait (ms)(milliseconds to wait=u32 1000) -> ()  [unwired: 1 out]
                    n132 = local write "Status"("Starting IV Sensor Scan" ("Status")) -> ()
                  }
                  frame #1 {
                    w673 = TRUE
                    n133 = while {
                      tunnel: w692 -> [w787]
                      tunnel: [w708] -> w690
                      tunnel: w693 -> [w781]
                      shift-right: [w784] -> w689
                      shift-left: w691 -> [w782]
                      tunnel: w688 -> [w778]
                      tunnel: [w777] -> w681
                      tunnel: [w776] -> w687
                      tunnel: [w770] -> w686
                      tunnel: w685 -> [w774]
                      tunnel: [w773] -> w684
                      tunnel: w683 -> [w772]
                      tunnel: w682 -> [w771]
                      tunnel: [w757] -> w677
                      tunnel: w680 -> [w756]
                      tunnel: w679 -> [w754]
                      tunnel: w678 -> [w753]
                      tunnel: w676 -> [w724]
                      tunnel: [w723] -> w675
                      shift-right: [w696] -> _
                      shift-left: w673 -> [w714]
                      shift-left: w673 -> [w716]
                      shift-left: w673 -> [w715]
                      tunnel: w674 -> [w707]
                      shift-left: w673 -> [w701]
                      shift-left: w673 -> [w700]
                      tunnel: w672 -> [w699]
                      tunnel: [w698] -> w671 mode=indexing
                      tunnel: [w694] -> w670
                      i -> [w775]
                      stop <- w764 continue-if-true
                      # "Change Bias Polarity\n+1 Chuck Bias\n-1  Pad bias"
                      # "Loop timing"
                      # "Plot Current"
                      n134 = Build Array(w714, w715, w716, w701, w700) -> (w713:bool[])
                      n135 = case shown="True" "Halt IV" {
                        selector: "Halt IV" -> [_ w793]
                        tunnel: [FALSE ("source") w796] -> w766
                        tunnel: w704 -> [_ w791]
                        frame #0 {
                        }
                        frame #1 {
                          n136 = flat-sequence {
                            tunnel: w793 -> [w799]
                            tunnel: [w799] -> w794
                            tunnel: w791 -> [w797]
                            tunnel: [w797] -> w789
                            tunnel: [w801] -> w795
                            tunnel: w794 -> [w802]
                            tunnel: [w800] -> w790
                            tunnel: w789 -> [w800]
                            tunnel: w795 -> [w805]
                            tunnel: [w805] -> w792
                            tunnel: w790 -> [w803]
                            tunnel: [w807] -> w796
                            tunnel: w792 -> [w807]
                            frame #0 {
                              n137 = call "Keith 237 Operate/Standby.vi"("source"=FALSE, "GPIB address"=w797) -> ()  [unwired: 1 in, 1 out]
                            }
                            frame #1 {
                              n138 = call "Prompt User for Input"("Enable"=w802) -> ("Yes"=w801:bool)  [unwired: 17 in, 1 out]
                            }
                            frame #2 {
                              n139 = call "Keith 237 Operate/Standby.vi"("source"=TRUE, "GPIB address"=w803) -> ()  [unwired: 1 in, 1 out]
                            }
                            frame #3 {
                              n140 = Wait (ms)(milliseconds to wait=750) -> ()  [unwired: 1 out]
                            }
                          }
                        }
                      }
                      n141 = Multiply(x=w781, y=w775) -> (x*y=w768:i32)
                      n142 = Multiply(x=w699, y=w768) -> (x*y=w755:dbl)
                      n143 = Equal To 0?(x=w775) -> (x = 0?=w762:bool)
                      n144 = flat-sequence {
                        tunnel: w753 -> [w811]
                        tunnel: w754 -> [w812]
                        tunnel: w782 -> [w813]
                        tunnel: [w813] -> w746
                        tunnel: [w812] -> w745
                        tunnel: [w811] -> w744
                        tunnel: [w810] -> w729
                        tunnel: w724 -> [w809]
                        tunnel: w707 -> [w808]
                        tunnel: [w808] -> w706
                        tunnel: w755 -> [w818]
                        tunnel: [w820] -> w752
                        tunnel: [w817] -> w751
                        tunnel: [w816] -> w750
                        tunnel: w746 -> [w819]
                        tunnel: w745 -> [w817]
                        tunnel: w744 -> [w816]
                        tunnel: [w815] -> w730
                        tunnel: w729 -> [w815]
                        tunnel: [w814] -> w709
                        tunnel: w706 -> [w814]
                        tunnel: w752 -> [w826]
                        tunnel: w751 -> [w825]
                        tunnel: w750 -> [w824]
                        tunnel: [w826] -> w749
                        tunnel: [w825] -> w748
                        tunnel: [w824] -> w747
                        tunnel: w730 -> [w823]
                        tunnel: [w822] -> w727
                        tunnel: [w821] -> w710
                        tunnel: w709 -> [w821]
                        tunnel: w749 -> [w829]
                        tunnel: w748 -> [w832]
                        tunnel: w747 -> [w831]
                        tunnel: [w828] -> w743
                        tunnel: [w832] -> w742
                        tunnel: [w831] -> w741
                        tunnel: [w830] -> w728
                        tunnel: w727 -> [w830]
                        tunnel: [w827] -> w711
                        tunnel: w710 -> [w827]
                        tunnel: w743 -> [w838]
                        tunnel: w742 -> [w837]
                        tunnel: w741 -> [w836]
                        tunnel: [w838] -> w740
                        tunnel: [w837] -> w739
                        tunnel: [w836] -> w738
                        tunnel: w728 -> [w835]
                        tunnel: [w834] -> w725
                        tunnel: [w833] -> w712
                        tunnel: w711 -> [w833]
                        tunnel: w740 -> [w849]
                        tunnel: w739 -> [w846]
                        tunnel: w738 -> [w845]
                        tunnel: [w839] -> w737
                        tunnel: [w841] -> w736
                        tunnel: [w840] -> w735
                        tunnel: [w844] -> w732
                        tunnel: [w843] -> w726
                        tunnel: w725 -> [w843]
                        tunnel: w712 -> [w842]
                        tunnel: [w842] -> w708
                        tunnel: [w842] -> w705
                        tunnel: [w839] -> w697
                        tunnel: w737 -> [w856]
                        tunnel: w736 -> [w855]
                        tunnel: w735 -> [w854]
                        tunnel: [w856] -> w734
                        tunnel: [w855] -> w733
                        tunnel: [w854] -> w702
                        tunnel: [w853] -> w731
                        tunnel: w732 -> [w853]
                        tunnel: w726 -> [w852]
                        tunnel: [w851] -> w723
                        tunnel: w705 -> [w850]
                        tunnel: [w850] -> w704
                        frame #0 {
                          n145 = call <vilib>:"Acquire Semaphore.vi"("semaphore"=w809) -> ("semaphore out"=w810:T1)  [unwired: 4 in, 2 out]
                        }
                        frame #1 {
                          n146 = call "Kei237_Set_Volt.vi"("Voltage"=w818, "error in"=w819, "GPIB"=w814) -> ("error out"=w820:errorcluster)
                        }
                        frame #2 {
                          n147 = call <vilib>:"Release Semaphore.vi"("semaphore"=w823) -> ("semaphore out"=w822:T1)  [unwired: 5 in, 1 out]
                        }
                        frame #3 {
                          n148 = call "Time Delay4"("error in (no error)"=w829) -> ("error out"=w828:errorcluster)  [unwired: 10 in]
                        }
                        frame #4 {
                          n149 = call <vilib>:"Acquire Semaphore.vi"("semaphore"=w835) -> ("semaphore out"=w834:T1)  [unwired: 4 in, 2 out]
                        }
                        frame #5 {
                          # "14"
                          # "10"
                          n150 = call "K237-read-current-2.vi"("error in"=w849, "GPIB"=w842) -> ("error out"=w848:T2, "Current"=w839:dbl)
                          n151 = call "KE6485 Read.vi"("error in (no error)"=w848, "instrument handle"=w846) -> ("error out"=w847:errorcluster, "reading"=w841:dbl)  [unwired: 7 in, 1 out]
                          n152 = call "KE6485 Read.vi"("error in (no error)"=w847, "instrument handle"=w845) -> ("error out"=w844:errorcluster, "reading"=w840:dbl)  [unwired: 7 in, 1 out]
                        }
                        frame #6 {
                          n153 = call <vilib>:"Release Semaphore.vi"("semaphore"=w852) -> ("semaphore out"=w851:T1)  [unwired: 5 in, 1 out]
                        }
                      }
                      n154 = local write "K237_Bias"(w755) -> ()
                      n155 = local read "voltage \ncompliance cutoff"() -> (w703:dbl)
                      n156 = Absolute Value(x=w697) -> (abs(x)=w695:dbl)
                      n157 = Absolute Value(x=w755) -> (abs(x)=w758:dbl)
                      n158 = Less?(x=w695, y=w703) -> (x < y?=w696:bool)
                      n159 = Not(x=w766) -> (.not. x?=w765:bool)
                      n160 = Wait Until Next ms Multiple(millisecond multiple=u32 1000) -> ()  [unwired: 1 out]
                      n161 = Select(t=w758, s=w756, f=w755) -> (s? t:f=w757:dbl)
                      n162 = Absolute Value(x=w757) -> (abs(x)=w722:dbl)
                      n163 = Absolute Value(x=w787) -> (abs(x)=w763:i32)
                      n164 = Or Array Elements(Boolean array=w713) -> (logical OR=w717:bool)
                      n165 = Less?(x=w722, y=w763) -> (x < y?=w767:bool)
                      n166 = Absolute Value(x=w734) -> (abs(x)=w761:dbl)
                      n167 = Absolute Value(x=w733) -> (abs(x)=w760:dbl)
                      n168 = Absolute Value(x=w702) -> (abs(x)=w759:dbl)
                      n169 = Compound Arithmetic op=AND(w717, w767, w765) -> (w764:bool)
                      n170 = Select(t=w761, s=w756, f=w734) -> (s? t:f=w721:dbl)
                      n171 = Select(t=w760, s=w756, f=w733) -> (s? t:f=w719:dbl)
                      n172 = Select(t=w759, s=w756, f=w702) -> (s? t:f=w720:dbl)
                      n173 = call "Total Current"("error in (no error)"=w731, "Reset"=w762, "Y Input"=w721, "X Input"=w757) -> ("error out"=w784:errorcluster, "XY Graph"=w770:cluster{"Y":dbl[], "Y":dbl[]}[])  [unwired: 1 in, 5 out]
                      "Total Current" <- w770
                      n174 = call "6485 Top"("error in (no error)"=w731, "Reset"=w762, "Y Input"=w719, "X Input"=w757) -> ("error out"=→"error out 5":errorcluster, "XY Graph"=w776:cluster{"Y":dbl[], "Y":dbl[]}[])  [unwired: 1 in, 5 out]
                      "6485 GRD (GPIB 10)" <- w776
                      n175 = call "6485 Bottom"("error in (no error)"=w731, "Reset"=w762, "Y Input"=w720, "X Input"=w757) -> ("error out"=→"error out 4":errorcluster, "XY Graph"=w777:cluster{"Y":dbl[], "Y":dbl[]}[])  [unwired: 1 in, 5 out]
                      "6485 ACTIVE (GPIB 14)" <- w777
                      n176 = Build Array(w757, w721, w720, w719) -> (w698:dbl[])
                      n177 = call-poly <vilib>:"Write To Spreadsheet File.vi"("delimiter (\\t)"="," ("delimiter (\\t)"), "format (%.3f)"="%.3e" ("file format"), "append to file? (new file:F)"=TRUE ("transpose? (no:F)"), "1D data"=w698, "file path (dialog if empty)"=w778) -> ("new file path (Not A Path if cancelled)"=w694:path)  [unwired: 2 in, 1 out]
                      n178 = call "XML_Data.vi"("Data Input Array"=w698, "Data Tag Names Array"=w772, "XML File Path"=w771, "DOM document in"=w774) -> ("DOM document out"=w773:refnum<k20>)  [unwired: 6 in, 1 out]
                    }
                  }
                  frame #2 {
                    n179 = local read "voltage \ncompliance level"() -> (w875:dbl)
                    n180 = local read "Bias Polarity"() -> (w872:dbl)
                    n181 = local read "IV-V-Steps"() -> (w873:i32)
                    n182 = local read "IV-V-Limit"() -> (w874:i32)
                    n183 = local read "Site # IV"() -> (w876:dbl)
                    n184 = Number To Fractional String(number=w876) -> (F-format string=w871:string)  [unwired: 3 in]
                    n185 = Number To Exponential String(number=w875) -> (E-format string=w870:string)  [unwired: 3 in]
                    n186 = Number To Fractional String(number=w872) -> (F-format string=w869:string)  [unwired: 3 in]
                    n187 = Number To Fractional String(number=w873) -> (F-format string=w868:string)  [unwired: 3 in]
                    n188 = Number To Fractional String(number=w874) -> (F-format string=w867:string)  [unwired: 3 in]
                    n189 = Build Array("K237 Parameters" ("string"), "Site Number" ("string"), "Voltage Compliance Level" ("string"), "Bias Polarity" ("string"), "Voltage Steps" ("string"), "Voltage Limit" ("string")) -> (w859:string[])
                    n190 = Build Array("", w871, w870, w869, w868, w867) -> (w858:string[])
                    n191 = Build Array(w859, w858) -> (w857:string[][])
                    n192 = call "Manual CV paramter_append.vi"("Array"=w857, "Path"=w877) -> ()  [unwired: 9 in, 1 out]
                  }
                  frame #3 {
                    n193 = call "IV_Sensor_Check.vi"("Data"=w910, "Titles"=w909) -> ("Boolean Pass/Fail Array"=w887:bool[], "Test Check Names"=w889:string[])  [unwired: 8 in]
                    n194 = Index Array(array=w889, index=0) -> (element=w908:string)
                    n195 = Index Array(array=w889, index=1) -> (element=w902:string)
                    n196 = Index Array(array=w889, index=2) -> (element=w901:string)
                    n197 = Index Array(array=w889, index=3) -> (element=w900:string)
                    n198 = Index Array(array=w889, index=4) -> (element=w899:string)
                    n199 = property on="Boolean" class="Bool (strict)"("Caption.Text"=w908) -> ()  [unwired: 2 in, 2 out]
                    n200 = property on="Boolean 2" class="Bool (strict)"("Caption.Text"=w902) -> ()  [unwired: 2 in, 2 out]
                    n201 = property on="Boolean 3" class="Bool (strict)"("Caption.Text"=w901) -> ()  [unwired: 2 in, 2 out]
                    n202 = property on="Boolean 4" class="Bool (strict)"("Caption.Text"=w900) -> ()  [unwired: 2 in, 2 out]
                    n203 = property on="Boolean 5" class="Bool (strict)"("Caption.Text"=w899) -> ()  [unwired: 2 in, 2 out]
                    n204 = Index Array(array=w887, index=0) -> (element=w893:bool)
                    n205 = Index Array(array=w887, index=1) -> (element=w891:bool)
                    n206 = Index Array(array=w887, index=2) -> (element=w888:bool)
                    n207 = Index Array(array=w887, index=3) -> (element=w890:bool)
                    n208 = Index Array(array=w887, index=4) -> (element=w892:bool)
                    n209 = local write "Boolean"(w893) -> ()
                    n210 = local write "Boolean 2"(w891) -> ()
                    n211 = local write "Boolean 3"(w888) -> ()
                    n212 = local write "Boolean 4"(w890) -> ()
                    n213 = local write "Boolean 5"(w892) -> ()
                  }
                }
                n214 = Open/Create/Replace File(file path (use dialog)=w623, operation (0:open)=T5."replace or create", access (0:read/write)=enum16{"read/write", "read-only", "write-only"}."read/write") -> (refnum out=w628:refnum<file>)  [unwired: 1 in, 4 out]
                n215 = Refnum to Path(1:w628) -> (0:w627:path)
                n216 = call-poly <vilib>:"Write To Spreadsheet File.vi"("delimiter (\\t)"="," ("delimiter (\\t)"), "append to file? (new file:F)"=FALSE, "2D data"=w624, "file path (dialog if empty)"=w627) -> ("new file path (Not A Path if cancelled)"=w622:path)  [unwired: 4 in]
                n217 = local write "Running Conditional"(TRUE) -> ()
                n218 = for {
                  tunnel: w580 -> [w659] mode=indexing
                  tunnel: [w656] -> w579 mode=indexing
                  n219 = Select(t="Passed" ("element"), s=w659, f="Failed" ("element")) -> (s? t:f=w656:string)
                }
                n220 = local read "File Name"() -> (w585:string)
                n221 = Concatenate Strings(w585, "_Check.csv" ("string")) -> (w586:string)
                n222 = Strip Path(path=w577) -> (stripped path=w589:path)  [unwired: 1 out]
                n223 = Index Array(array=w614, index=0) -> (element=w613:string)
                n224 = Index Array(array=w614, index=1) -> (element=w612:string)
                n225 = Index Array(array=w614, index=2) -> (element=w611:string)
                n226 = Index Array(array=w614, index=3) -> (element=w610:string)
                n227 = Index Array(array=w614, index=4) -> (element=w609:string)
                n228 = property on="Tab Control 2" class="TabCtl (strict)"("Visible"=TRUE) -> ()  [unwired: 2 in, 2 out]
                n229 = Index Array(array=w579, index=0) -> (element=w603:string)
                n230 = Index Array(array=w579, index=1) -> (element=w602:string)
                n231 = Index Array(array=w579, index=2) -> (element=w601:string)
                n232 = Index Array(array=w579, index=3) -> (element=w600:string)
                n233 = Index Array(array=w579, index=4) -> (element=w599:string)
                n234 = Build Path(base path=w589, name or relative path=w586) -> (appended path=w588:path)
                n235 = Build Array(w613, w612, w611, w610, w609) -> (w598:string[])
                n236 = Build Array(w603, w602, w601, w600, w599) -> (w597:string[])
                n237 = Build Array(w585, "Passed/Failed" ("element")) -> (w582:string[])
                n238 = Build Array(w598, w597) -> (w596:string[][])
                n239 = Transpose 2D Array(2D array=w596) -> (transposed array=w581:string[][])
                n240 = Open/Create/Replace File(file path (use dialog)=w588, operation (0:open)=T5."replace or create", access (0:read/write)=enum16{"read/write", "read-only", "write-only"}."read/write") -> (refnum out=w594:refnum<file>)  [unwired: 1 in, 4 out]
                n241 = Refnum to Path(1:w594) -> (0:w591:path)
                n242 = Build Array (concatenate)(w582, w581) -> (w583:string[][])
                n243 = call-poly <vilib>:"Write To Spreadsheet File.vi"("delimiter (\\t)"="," ("delimiter (\\t)"), "append to file? (new file:F)"=FALSE, "2D data"=w583, "file path (dialog if empty)"=w591) -> ()  [unwired: 4 in, 1 out]
              }
              frame #1 {
                w919 = FALSE ("Boolean")
                w922 = cluster{"Y":dbl[], "Y":dbl[]}[] [] ("XY Graph")
                n244 = local write "Boolean"(w919) -> ()
                n245 = local write "Boolean 2"(w919) -> ()
                n246 = local write "Boolean 3"(w919) -> ()
                n247 = local write "Boolean 4"(w919) -> ()
                n248 = local write "Boolean 5"(w919) -> ()
              }
            }
            n249 = call-poly <vilib>:"Close.vi"("node"=w548) -> ()  [unwired: 8 in, 1 out]
          }
          frame #3 {
            w926 = FALSE
            n250 = case shown="True" w926 {
              tunnel: w931 -> [w936 w941]
              tunnel: [w936 w940] -> w930
              tunnel: [w935 w939] -> w929
              tunnel: w928 -> [_ w938]
              tunnel: w927 -> [w935 w937]
              frame #0 {
              }
              frame #1 {
                n251 = while {
                  tunnel: [w957] -> w939
                  tunnel: w941 -> [w951]
                  tunnel: [w951] -> w940
                  tunnel: w938 -> [w945]
                  tunnel: w937 -> [w942]
                  i -> [w956]
                  stop <- w953 continue-if-true
                  n252 = Multiply(x=400, y=w956) -> (x*y=w948:i32)
                  n253 = Sign(1:w945) -> (0:w950:dbl)
                  n254 = Subtract(x=w945, y=w948) -> (x-y=w947:dbl)
                  n255 = Add(x=w945, y=w948) -> (x+y=w946:dbl)
                  n256 = Greater Than 0?(x=w950) -> (x > 0?=w949:bool)
                  n257 = Select(t=w947, s=w949, f=w946) -> (s? t:f=w943:dbl)
                  n258 = Absolute Value(x=w943) -> (abs(x)=w944:dbl)
                  n259 = local write "K237_Bias"(w943) -> ()
                  n260 = call "Time Delay"("error in (no error)"=w942) -> ("error out"=w952:errorcluster)  [unwired: 10 in]
                  n261 = Greater?(x=w944, y=400) -> (0:w953:bool)
                  n262 = call "Kei237_Set_Volt.vi"("Voltage"=w943, "error in"=w952, "GPIB"=w951) -> ("error out"=w957:errorcluster)
                }
              }
            }
            n263 = local write "Running Conditional"(w926) -> ()
            n264 = local write "Running?"(w926) -> ()
          }
          frame #4 {
            n265 = Wait (ms)(milliseconds to wait=250) -> ()  [unwired: 1 out]
          }
          frame #5 {
            w964 = TRUE ("append to file? (new file:F)")
            w1005 = 0
            n266 = local read "Site Number"() -> (w975:i32)
            n267 = In Range and Coerce(upper limit=3, x=w1018, lower limit=0) -> (In Range?=w994:bool)  [unwired: 1 out]
            n268 = case shown="False" w994 {
              tunnel: [w1145 w1157] -> w1021
              tunnel: w1018 -> [w1144 _]
              frame #0 {
                n269 = In Range and Coerce(upper limit=11, x=w1144, lower limit=4) -> (In Range?=w1146:bool)  [unwired: 1 out]
                n270 = case shown="False" w1146 {
                  tunnel: [w1153 w1156] -> w1145
                  tunnel: w1144 -> [w1150 _]
                  frame #0 {
                    n271 = In Range and Coerce(upper limit=17, x=w1150, lower limit=12) -> (In Range?=w1149:bool)  [unwired: 1 out]
                    n272 = case shown="False" w1149 {
                      tunnel: [w1154 w1155] -> w1153
                      frame #0 {
                        w1154 = 3
                        n273 = property on="Archive" class="TabCtl (strict)"("Value"=w1154) -> ()  [unwired: 2 in, 2 out]
                      }
                      frame #1 {
                        w1155 = 1
                        n274 = property on="Archive" class="TabCtl (strict)"("Value"=w1155) -> ()  [unwired: 2 in, 2 out]
                      }
                    }
                  }
                  frame #1 {
                    w1156 = 2
                    n275 = property on="Archive" class="TabCtl (strict)"("Value"=w1156) -> ()  [unwired: 2 in, 2 out]
                  }
                }
              }
              frame #1 {
                w1157 = 0
                n276 = property on="Archive" class="TabCtl (strict)"("Value"=w1157) -> ()  [unwired: 2 in, 2 out]
              }
            }
            n277 = local write "Status"("IV Sensor Scan Finished" ("Status")) -> ()
            n278 = case shown="1, Default" w975 {
              tunnel: ["D_BL_" "D_TL_" "D_TR_" "D_BR_" "L_TT_" "L_FL_" "L_LL_" "L_CL_" "L_CR_" "L_RR_" "L_FR_" "L_BB_" "S_TL_" "S_TR_" "S_CL_" "S_CR_" "S_BL_" "S_BR_" "A_TL_" "A_TR_" "A_BL_" "A_BR_"] -> w974
              tunnel: ["Diode" "Diode" "Diode" "Diode" w1038 w1044 w1050 w1056 w1062 w1068 w1074 w1080 w1086 w1092 w1098 w1104 w1110 w1116 w1122 w1129 w1135 w1141] -> _
              tunnel: ["D1" "D2" "D3" "D4" "L5-2x8" "L6-2x8" "L7-2x8" "L8-2x8" "L9-2x8" "L10-2x8" "L11-2x8" "L12-2x8" "S13-1x1" "S14-1x1" "S15-1x1" "S16-1x1" "S17-1x1" "S18-1x1" "SE19" "SE20" "SE21" "SE22"] -> _
              frame #0 {
              }
              frame #1 {
              }
              frame #2 {
              }
              frame #3 {
              }
              frame #4 {
                n279 = call <vilib>:"Space Constant.vi"() -> ("String"=w1040:string)
                n280 = Concatenate Strings("2x8", w1040, "X") -> (w1038:string)
              }
              frame #5 {
                n281 = call <vilib>:"Space Constant.vi"() -> ("String"=w1046:string)
                n282 = Concatenate Strings("2x8", w1046, "FMM") -> (w1044:string)
              }
              frame #6 {
                n283 = call <vilib>:"Space Constant.vi"() -> ("String"=w1052:string)
                n284 = Concatenate Strings("2x8", w1052, "FMM") -> (w1050:string)
              }
              frame #7 {
                n285 = call <vilib>:"Space Constant.vi"() -> ("String"=w1058:string)
                n286 = Concatenate Strings("2x8", w1058, "Close") -> (w1056:string)
              }
              frame #8 {
                n287 = call <vilib>:"Space Constant.vi"() -> ("String"=w1064:string)
                n288 = Concatenate Strings("2x8", w1064, "X") -> (w1062:string)
              }
              frame #9 {
                n289 = call <vilib>:"Space Constant.vi"() -> ("String"=w1070:string)
                n290 = Concatenate Strings("2x8", w1070, "FM") -> (w1068:string)
              }
              frame #10 {
                n291 = call <vilib>:"Space Constant.vi"() -> ("String"=w1076:string)
                n292 = Concatenate Strings("2x8", w1076, "FM") -> (w1074:string)
              }
              frame #11 {
                n293 = call <vilib>:"Space Constant.vi"() -> ("String"=w1082:string)
                n294 = Concatenate Strings("2x8", w1082, "Close") -> (w1080:string)
              }
              frame #12 {
                n295 = call <vilib>:"Space Constant.vi"() -> ("String"=w1088:string)
                n296 = Concatenate Strings("1x1", w1088, "FMM") -> (w1086:string)
              }
              frame #13 {
                n297 = call <vilib>:"Space Constant.vi"() -> ("String"=w1094:string)
                n298 = Concatenate Strings("1x1", w1094, "FMM") -> (w1092:string)
              }
              frame #14 {
                n299 = call <vilib>:"Space Constant.vi"() -> ("String"=w1100:string)
                n300 = Concatenate Strings("1x1", w1100, "Close") -> (w1098:string)
              }
              frame #15 {
                n301 = call <vilib>:"Space Constant.vi"() -> ("String"=w1106:string)
                n302 = Concatenate Strings("1x1", w1106, "FM") -> (w1104:string)
              }
              frame #16 {
                n303 = call <vilib>:"Space Constant.vi"() -> ("String"=w1112:string)
                n304 = Concatenate Strings("1x1", w1112, "X") -> (w1110:string)
              }
              frame #17 {
                n305 = call <vilib>:"Space Constant.vi"() -> ("String"=w1118:string)
                n306 = Concatenate Strings("1x1", w1118, "FMM") -> (w1116:string)
              }
              frame #18 {
                n307 = call <vilib>:"Space Constant.vi"() -> ("String"=w1124:string)
                n308 = Concatenate Strings("Slim-Edge", w1124, "FMM_S3") -> (w1122:string)
              }
              frame #19 {
                n309 = call <vilib>:"Space Constant.vi"() -> ("String"=w1130:string)
                n310 = Concatenate Strings("Slim-Edge", w1130, "FMM_S3") -> (w1129:string)
              }
              frame #20 {
                n311 = call <vilib>:"Space Constant.vi"() -> ("String"=w1136:string)
                n312 = Concatenate Strings("Slim-Edge", w1136, "FMM_S3") -> (w1135:string)
              }
              frame #21 {
                n313 = call <vilib>:"Space Constant.vi"() -> ("String"=w1142:string)
                n314 = Concatenate Strings("Slim-Edge", w1142, "FMM_S3") -> (w1141:string)
              }
            }
            n315 = call "Kei237_Set_Volt.vi"("Voltage"=w1005, "error in"=w1023, "GPIB"=w986) -> ("error out"=w987:errorcluster)
            n316 = local write "K237_Bias"(w1005) -> ()
            n317 = local read "Wafer Number"() -> (w972:string)
            n318 = Unbundle(w1004) -> (w1003:cluster{"Y":dbl[], "Y":dbl[]}[], w1002:cluster{"Y":dbl[], "Y":dbl[]}[], w995:cluster{"Y":dbl[], "Y":dbl[]}[], w1001:cluster{"Y":dbl[], "Y":dbl[]}[], w1000:cluster{"Y":dbl[], "Y":dbl[]}[], w999:cluster{"Y":dbl[], "Y":dbl[]}[], w998:cluster{"Y":dbl[], "Y":dbl[]}[], w997:cluster{"Y":dbl[], "Y":dbl[]}[], w996:cluster{"Y":dbl[], "Y":dbl[]}[], w991:cluster{"Y":dbl[], "Y":dbl[]}[], w992:cluster{"Y":dbl[], "Y":dbl[]}[], w993:cluster{"Y":dbl[], "Y":dbl[]}[])
            n319 = call "Keith 237 Operate/Standby.vi"("source"=FALSE, "error in"=w987, "GPIB address"=w986) -> ("error out"=w984:T2)
            n320 = Concatenate Strings("W" ("string"), w974, w972) -> (w970:string)
            n321 = case shown="0, Default" w1021 {
              tunnel: w1017 -> [w1175 w1193 w1211 w1229]
              tunnel: w1016 -> [w1174 w1192 w1210 w1228]
              tunnel: w1015 -> [w1173 w1191 w1209 w1227]
              tunnel: [w1163 w1189 w1206 w1226] -> w1014
              tunnel: [w1161 w1187 w1207 w1225] -> w1013
              tunnel: [w1162 w1188 w1208 w1224] -> w1012
              tunnel: w1003 -> [w1172 w1189 w1206 w1226]
              tunnel: w1002 -> [w1171 w1187 w1207 w1225]
              tunnel: w995 -> [w1170 w1188 w1208 w1224]
              tunnel: [w1169 w1186 w1205 w1223] -> w1011
              tunnel: [w1164 w1179 w1199 w1218] -> w1010
              tunnel: [w1166 w1183 w1204 w1222] -> w1009
              tunnel: w1001 -> [w1169 w1190 w1205 w1223]
              tunnel: w996 -> [w1164 w1179 w1201 w1218]
              tunnel: w1000 -> [w1166 w1185 w1204 w1222]
              tunnel: [w1168 w1182 w1203 w1221] -> w1008
              tunnel: [w1165 w1181 w1197 w1220] -> w1007
              tunnel: [w1167 w1180 w1198 w1219] -> w1006
              tunnel: w999 -> [w1168 w1184 w1203 w1221]
              tunnel: w998 -> [w1165 w1181 w1202 w1220]
              tunnel: w997 -> [w1167 w1180 w1200 w1219]
              tunnel: w993 -> [w1158 w1176 w1194 w1216]
              tunnel: w992 -> [w1159 w1177 w1195 w1215]
              tunnel: w991 -> [w1160 w1178 w1196 w1217]
              tunnel: [w1160 w1178 w1196 w1214] -> w990
              tunnel: [w1159 w1177 w1195 w1213] -> w989
              tunnel: [w1158 w1176 w1194 w1212] -> w988
              frame #0 {
                # "Diodes"
                n322 = Insert Into Array(array=w1172, new element=w1175) -> (w1163:cluster{"Y":dbl[], "Y":dbl[]}[])  [unwired: 1 in]
                "Diode ACTIVE Archive" <- w1163
                n323 = Insert Into Array(array=w1171, new element=w1174) -> (w1161:cluster{"Y":dbl[], "Y":dbl[]}[])  [unwired: 1 in]
                "Diode GRD Archive" <- w1161
                n324 = Insert Into Array(array=w1170, new element=w1173) -> (w1162:cluster{"Y":dbl[], "Y":dbl[]}[])  [unwired: 1 in]
                "Diode Total Current Archive" <- w1162
              }
              frame #1 {
                # "Single Chips"
                n325 = Insert Into Array(array=w1190, new element=w1193) -> (w1186:cluster{"Y":dbl[], "Y":dbl[]}[])  [unwired: 1 in]
                "Single Chip ACTIVE Archive" <- w1186
                n326 = Insert Into Array(array=w1185, new element=w1192) -> (w1183:cluster{"Y":dbl[], "Y":dbl[]}[])  [unwired: 1 in]
                "Single Chip GRD Archive" <- w1183
                n327 = Insert Into Array(array=w1184, new element=w1191) -> (w1182:cluster{"Y":dbl[], "Y":dbl[]}[])  [unwired: 1 in]
                "Single Chip Total Current Archive" <- w1182
              }
              frame #2 {
                # "2x8s"
                n328 = Insert Into Array(array=w1202, new element=w1211) -> (w1197:cluster{"Y":dbl[], "Y":dbl[]}[])  [unwired: 1 in]
                "2x8 ACTIVE Archive" <- w1197
                n329 = Insert Into Array(array=w1200, new element=w1210) -> (w1198:cluster{"Y":dbl[], "Y":dbl[]}[])  [unwired: 1 in]
                "2x8 GRD Archive" <- w1198
                n330 = Insert Into Array(array=w1201, new element=w1209) -> (w1199:cluster{"Y":dbl[], "Y":dbl[]}[])  [unwired: 1 in]
                "2x8 Total Current Archive" <- w1199
              }
              frame #3 {
                # "Slim-Edge"
                n331 = Insert Into Array(array=w1217, new element=w1229) -> (w1214:cluster{"Y":dbl[], "Y":dbl[]}[])  [unwired: 1 in]
                "Slim-Edge ACTIVE Archive" <- w1214
                n332 = Insert Into Array(array=w1215, new element=w1228) -> (w1213:cluster{"Y":dbl[], "Y":dbl[]}[])  [unwired: 1 in]
                "Slim-Edge GRD Archive" <- w1213
                n333 = Insert Into Array(array=w1216, new element=w1227) -> (w1212:cluster{"Y":dbl[], "Y":dbl[]}[])  [unwired: 1 in]
                "Slim-Edge Total Current Archive" <- w1212
              }
            }
            n334 = local read "Contact Check Result"() -> (w976:string)
            n335 = Wait Until Next ms Multiple(millisecond multiple=u32 250) -> ()  [unwired: 1 out]
            n336 = local read "Contact Check"() -> (w982:bool)
            n337 = Equal?(x=w976, y="Skipped" ("Contact Check Result")) -> (x = y?=w978:bool)
            n338 = Select(t="Passed", s=w982, f="Failed") -> (s? t:f=w979:string)
            n339 = Select(t=w976, s=w978, f=w979) -> (s? t:f=w971:string)
            n340 = Build Array(w970) -> (w967:string[])
            n341 = Build Array(w971) -> (w966:string[])
            n342 = Build Array(w967, w966) -> (w965:string[][])
            n343 = call-poly <vilib>:"Write To Spreadsheet File.vi"("delimiter (\\t)"="," ("delimiter (\\t)"), "transpose? (no:F)"=w964, "append to file? (new file:F)"=w964, "2D data"=w965, "file path (dialog if empty)"=w968) -> ()  [unwired: 3 in, 1 out]
          }
        }
        n344 = call "Auto_IV_CV_XML_Excell_Label.vi"("Cluster"=w165, "Loop Count"=w166, "IV or CV"=w167) -> ("File Name"=w163:string, "Excell Cell Title"=w162:string[], "XML Data Tags"=w164:string[])  [unwired: 6 in]
        "File Name" <- w163
        n345 = Build Array("Bias", "Total", "Active", "Guardring") -> (w161:string[])
        n346 = Concatenate Strings(w163, "_IV.csv" ("string")) -> (w212:string)
        n347 = Concatenate Strings(w163, "_IV.xml" ("string")) -> (w210:string)
        n348 = Build Array("VOLTAGE_VOLT", "TOT_CURRENT_AMP", "ACTV_CURRENT_AMP", "GRD_CURRENT_AMP") -> (w169:string[])
        n349 = Build Path(base path=w202, name or relative path=w212) -> (appended path=w140:path)
        n350 = Build Path(base path=w141, name or relative path=w210) -> (appended path=w209:path)
        n351 = Build Array(w162, w161) -> (w160:string[][])
        n352 = call "XML_Initilize.vi"("User Input"=w164) -> ("DOM document out"=w218:refnum<k20>)  [unwired: 10 in]
      }
      n353 = call "KE6485 Close.vi"("error in (no error)"=w125, "instrument handle"=refnum<k15> "GPIB0::10::INSTR") -> ("error out"=w128:errorcluster)  [unwired: 9 in]
      n354 = call "KE6485 Close.vi"("error in (no error)"=w128, "instrument handle"=refnum<k15> "GPIB0::14::INSTR") -> ("error out"=w124:errorcluster)  [unwired: 9 in]
      n355 = call "Keith 237 Reset.vi"("GPIB address"=w137, "error in"=w124) -> ("error out"=w129:T2)
    }
    frame #2 {
      n356 = Wait (ms)(milliseconds to wait=u32 500) -> ()  [unwired: 1 out]
    }
    frame #3 {
      n357 = Build Array(16, 10, 14) -> (w1241:i32[])
      n358 = EnableLocal(2:w1237, 3:w1241, 4:0) -> (0:w1236:errorcluster)  [unwired: 1 out]
      n359 = local write "Status"("Full IV Scan Finished" ("Status")) -> ()
    }
    frame #4 {
      # "Ask the operator to\nchange the wires \nfrom IV to CV"
      n360 = call "RE-WIRE  from IV to CV"("Enable"=TRUE) -> ("OK"=w1244:bool)  [unwired: 17 in, 1 out]
      n361 = local read "semaphore"() -> (w1242:T1)
      n362 = Not(x=w1244) -> (.not. x?=w1245:bool)
      n363 = local write "IV or CV"(1 ("IV or CV")) -> ()
      n364 = Stop(stop? (T)=w1245) -> ()
    }
    frame #5 {
      w1250 = u16 5 items=["auto / auto", "1 nA / 1.1 V", "10 nA / 11 V", "100 nA / 110 V", "0.001 mA / 1100 V", "0.01 mA / 1100 V", "0.1 mA / 1100 V", "1 mA / 1100 V", "10 mA / 1100 V", "100 mA / 1100 V"] ("compliance/\nmeasurement range (auto:0)")
      w1265 = 1e-05 ("current \ncompliance level")
      w1261 = u16 5 items=["auto / auto", "1 nA / 1.1 V", "10 nA / 11 V", "100 nA / 110 V", "0.001 mA / 1100 V", "0.01 mA / 1100 V", "0.1 mA / 1100 V", "1 mA / 1100 V", "10 mA / 1100 V", "100 mA / 1100 V"] ("source range\nI source / V source (auto:0)")
      w1266 = u16 0 items=["voltage/current", "current/voltage"] ("source/measure (V/I:0)")
      w1267 = u16 0 items=["DC", "sweep"] ("function (DC:0)")
      w1253 = "16" ("GPIB address")
      w1269 = 1000.0 ("Time Delay mS")
      w1271 = TRUE ("reset")
      w1275 = 0.5  # Voltage Level
      w1276 = 5.0 ("Number of Averages")
      w1277 = 10000.0 ("Frequency")
      w1278 = u16 7 items=["None", "Cs", "Cp", "Ls", "Lp", "Rs", "Rp", "DF", "Q", "Z", "Y", "Phase", "ESR", "Gp", "Xs", "Bp"] ("Secondary Parameter")
      w1279 = u16 2 items=["AUTO", "Cs", "Cp", "Ls", "Lp", "Rs", "Rp", "DF", "Q", "Z", "Y", "Phase", "ESR", "Gp", "Xs", "Bp"] ("Primary Parameter")
      w1280 = u16 0 items=["Voltage", "Current"] ("Signal Type")
      w1281 = u16 0 items=["Measured", "Deviation", "% Deviation", "No Display"] ("Display")
      w1282 = u16 2 items=["Off", "Internal", "External"] ("Bias")
      n365 = DevClear(2:w1255, 3:i16 16 ("address"), 4:0) -> (0:w1257:errorcluster)  [unwired: 1 out]
      n366 = call "Keith 237 Basic Config.vi"("GPIB address"=w1253, "source/measure (V/I:0)"=w1266, "function (DC:0)"=w1267, "source range\nI source / V source (auto:0)"=w1261, "source level"=0.0, "error in"=w1257, "1100 V range (disabled:F)"=TRUE, "current \ncompliance level"=w1265, "compliance/\nmeasurement range (auto:0)"=w1250) -> ("error out"=w1264:T2)  [unwired: 10 in]
      n367 = call "Keith 237 Operate/Standby.vi"("source"=FALSE, "error in"=w1264, "GPIB address"=w1253) -> ("error out"=w1262:T2)
      n368 = local write "Status"("Setting CV Scan Parameters" ("Status")) -> ()
      n369 = call "Keith 237 Send Trigger.vi"("GPIB address"=w1253, "error in"=w1262) -> ("error out"=w1256:T2)
      n370 = call "7000 Series Initialize.vi"("error in (no error)"=w1256, "reset"=w1271, "ID query"=w1271, "instrument descriptor"="GPIB::4") -> ("error out"=w1283:errorcluster, "Identification"=→"QuadTech Status":string, "VISA session"=w1272:refnum<visa-resource-name>)
      n371 = call "7000 Series Configure.vi"("inst handle in"=w1272, "Primary Parameter"=w1279, "Secondary Parameter"=w1278, "Frequency"=w1277, "Number of Averages"=w1276, "error in"=w1283, "Bias"=w1282, "Display"=w1281, "Signal Type"=w1280, "Optional"="CONF:SWE:SWE OFF", "Time Delay mS"=w1269, "Voltage Level"=w1275) -> ("inst handle out"=w1254:refnum<visa-resource-name>, "Identification"=w1273:string, "error out"=w1252:T8)  [unwired: 13 in]
      n372 = local write "QuadTech Status"(w1273) -> ()
      "Frequency" <- w1277
      "Voltage Level" <- w1275
      "Number of Averages" <- w1276
      "Time Delay mS" <- w1269
      "Primary Parameter" <- w1279
      "Auto Compliance" <- w1265
      "Secondary Parameter" <- w1278
    }
    frame #6 {
      n373 = case shown="0, Default" w1286 {
        frame #0 {
          n374 = local read "Auto Compliance"() -> (w1291:dbl)
          n375 = Multiply(x=w1291, y=0.98) -> (x*y=w1290:dbl)
          n376 = local write "Compliance"(w1290) -> ()
        }
        frame #1 {
          n377 = Multiply(x=1e-09, y=0.98) -> (x*y=→"Compliance":dbl)
        }
        frame #2 {
          n378 = Multiply(x=1e-08, y=0.98) -> (x*y=w1296:dbl)
          n379 = local write "Compliance"(w1296) -> ()
        }
        frame #3 {
          n380 = Multiply(x=1e-07, y=0.98) -> (x*y=w1299:dbl)
          n381 = local write "Compliance"(w1299) -> ()
        }
        frame #4 {
          n382 = Multiply(x=1e-06, y=0.98) -> (x*y=w1302:dbl)
          n383 = local write "Compliance"(w1302) -> ()
        }
        frame #5 {
          n384 = Multiply(x=1e-05, y=0.98) -> (x*y=w1306:dbl)
          n385 = local write "Compliance"(w1306) -> ()
        }
        frame #6 {
          n386 = Multiply(x=0.0001, y=0.98) -> (x*y=w1308:dbl)
          n387 = local write "Compliance"(w1308) -> ()
        }
        frame #7 {
          n388 = Multiply(x=0.001, y=0.98) -> (x*y=w1312:dbl)
          n389 = local write "Compliance"(w1312) -> ()
        }
        frame #8 {
          n390 = Multiply(x=0.001, y=0.98) -> (x*y=w1314:dbl)
          n391 = local write "Compliance"(w1314) -> ()
        }
        frame #9 {
          n392 = Multiply(x=0.001, y=0.98) -> (x*y=w1317:dbl)
          n393 = local write "Compliance"(w1317) -> ()
        }
      }
    }
    frame #7 {
      w1334 = u16 0 items=["Off", "Internal", "External"] ("Bias")
      n394 = for {
        N: w1324 -> [_]
        tunnel: w1337 -> [w1402]
        tunnel: w1336 -> [w1401]
        tunnel: [w1372] -> w1332
        tunnel: [w1371] -> w1330
        shift-right: [w1399] -> w1331
        shift-left: w1335 -> [w1400]
        shift-right: [w1396] -> _
        shift-left: _ -> [w1368]
        shift-right: [w1395] -> _
        shift-left: _ -> [w1367]
        shift-right: [w1394] -> _
        shift-left: _ -> [w1366]
        tunnel: w1327 -> [w1380]
        tunnel: w1323 -> [w1364]
        tunnel: w1321 -> [w1344]
        tunnel: w1320 -> [w1338]
        i -> [w1345]
        # "User Input Array\nElement 0: Comment Description (XML_Header)\nElement 1: Serial Number\nElement 2: Kind of Part\nElement 3: User\nElement 4: Extension Table Name\nElement 5: Comment Description (XML_Data_Set)\nElement 6: Name (XML_Header)\nElement 7: Run Name (XML_Header)"
        # "XML Data Tags for CV scan"
        n395 = Increment(x=w1345) -> (x+1=→"Site # CV":i32)
        n396 = local read "IV or CV"() -> (w1346:i32)
        n397 = Bundle(w1368, w1367, w1366) -> (w1365:T9)  [unwired: 1 in]
        n398 = call "Auto_IV_CV_XML_Excell_Label.vi"("Cluster"=w1344, "Loop Count"=w1345, "IV or CV"=w1346) -> ("File Name"=w1342:string, "Excell Cell Title"=w1341:string[], "XML Data Tags"=w1343:string[])  [unwired: 6 in]
        n399 = flat-sequence {
          tunnel: [w1411] -> w1363
          tunnel: w1402 -> [w1411]
          tunnel: [w1410] -> w1362
          tunnel: w1401 -> [w1410]
          tunnel: [w1409] -> w1361
          tunnel: w1400 -> [w1409]
          tunnel: w1345 -> [w1405]
          tunnel: w1364 -> [w1407]
          tunnel: [w1407] -> w1360
          tunnel: [w1406] -> w1359
          tunnel: [w1405] -> w1349
          tunnel: [w1403] -> w1348
          tunnel: [w1457] -> w1393
          tunnel: [w1456] -> w1392
          tunnel: [w1455] -> w1391
          tunnel: [w1448] -> w1386
          tunnel: w1385 -> [w1447]
          tunnel: w1379 -> [w1446]
          tunnel: w1376 -> [w1445]
          tunnel: [w1443] -> w1375
          tunnel: w1348 -> [w1438]
          tunnel: w1349 -> [w1440]
          tunnel: w1359 -> [w1437]
          tunnel: w1360 -> [w1442]
          tunnel: w1361 -> [w1458]
          tunnel: w1362 -> [w1455]
          tunnel: w1363 -> [w1459]
          tunnel: w1340 -> [w1436]
          tunnel: w1339 -> [w1435]
          tunnel: w1393 -> [w1810]
          tunnel: [w1810] -> w1390
          tunnel: w1392 -> [w1809]
          tunnel: [w1809] -> w1389
          tunnel: w1391 -> [w1808]
          tunnel: [w1808] -> w1388
          tunnel: [w1807] -> w1387
          tunnel: w1386 -> [w1807]
          tunnel: w1375 -> [w1806]
          tunnel: [w1806] -> w1374
          tunnel: w1390 -> [w1815]
          tunnel: [w1814] -> w1358
          tunnel: w1389 -> [w1818]
          tunnel: [w1818] -> w1356
          tunnel: w1388 -> [w1817]
          tunnel: [w1816] -> w1354
          tunnel: w1387 -> [w1813]
          tunnel: w1374 -> [w1812]
          tunnel: [w1812] -> w1352
          tunnel: w1358 -> [w1846]
          tunnel: [w1846] -> w1357
          tunnel: w1356 -> [w1845]
          tunnel: [w1845] -> w1355
          tunnel: w1354 -> [w1844]
          tunnel: [w1844] -> w1353
          tunnel: w1352 -> [w1843]
          tunnel: [w1843] -> w1351
          tunnel: [w1869] -> w1372
          tunnel: [w1848] -> w1399
          tunnel: w1357 -> [w1868]
          tunnel: w1355 -> [w1869]
          tunnel: w1353 -> [w1850]
          tunnel: w1345 -> [w1852]
          tunnel: [w1861] -> w1396
          tunnel: [w1860] -> w1395
          tunnel: [w1859] -> w1394
          tunnel: w1351 -> [w1857]
          tunnel: [w1850] -> w1371
          tunnel: w1365 -> [w1856]
          frame #0 {
            n400 = Increment(x=w1405) -> (x+1=w1404:i32)
            n401 = case shown="1" w1404 {
              tunnel: [TRUE w1413 w1414 w1415 w1416 w1417 w1418 w1419 w1420 w1421 w1422 w1423 w1424 w1425 w1426 w1427 w1428 w1429 w1430 w1431 w1432 w1433 w1434] -> w1403
              frame #0 {
              }
              frame #1 {
                n402 = local read "Site 1"() -> (w1413:bool)
              }
              frame #2 {
                n403 = local read "Site 2"() -> (w1414:bool)
              }
              frame #3 {
                n404 = local read "Site 3"() -> (w1415:bool)
              }
              frame #4 {
                n405 = local read "Site 4"() -> (w1416:bool)
              }
              frame #5 {
                n406 = local read "Site 5"() -> (w1417:bool)
              }
              frame #6 {
                n407 = local read "Site 6"() -> (w1418:bool)
              }
              frame #7 {
                n408 = local read "Site 7"() -> (w1419:bool)
              }
              frame #8 {
                n409 = local read "Site 8"() -> (w1420:bool)
              }
              frame #9 {
                n410 = local read "Site 9"() -> (w1421:bool)
              }
              frame #10 {
                n411 = local read "Site 10"() -> (w1422:bool)
              }
              frame #11 {
                n412 = local read "Site 11"() -> (w1423:bool)
              }
              frame #12 {
                n413 = local read "Site 12"() -> (w1424:bool)
              }
              frame #13 {
                n414 = local read "Site 13"() -> (w1425:bool)
              }
              frame #14 {
                n415 = local read "Site 14"() -> (w1426:bool)
              }
              frame #15 {
                n416 = local read "Site 15"() -> (w1427:bool)
              }
              frame #16 {
                n417 = local read "Site 16"() -> (w1428:bool)
              }
              frame #17 {
                n418 = local read "Site 17"() -> (w1429:bool)
              }
              frame #18 {
                n419 = local read "Site 18"() -> (w1430:bool)
              }
              frame #19 {
                n420 = local read "Site 19"() -> (w1431:bool)
              }
              frame #20 {
                n421 = local read "Site 20"() -> (w1432:bool)
              }
              frame #21 {
                n422 = local read "Site 21"() -> (w1433:bool)
              }
              frame #22 {
                n423 = local read "Site 22"() -> (w1434:bool)
              }
            }
            n424 = call "Skip Current Subsite2"("Enable"=w1403) -> ("Skip Subsite"=w1406:bool)  [unwired: 17 in, 1 out]
            n425 = Wait (ms)(milliseconds to wait=u32 250) -> ()  [unwired: 1 out]
          }
          frame #1 {
            n426 = Not(x=w1438) -> (.not. x?=w1439:bool)
            n427 = Or(x=w1439, y=w1437) -> (x .or. y?=w1441:bool)
            n428 = case shown="False" w1441 {
              tunnel: "CV-V-Limit" -> [w1512 _]
              tunnel: "CV-V-Steps" -> [w1511 _]
              tunnel: w1459 -> [w1510 w1802]
              tunnel: w1458 -> [w1509 w1801]
              tunnel: [w1508 w1801] -> w1457
              tunnel: [w1507 w1802] -> w1456
              tunnel: w1455 -> [w1506 _]
              tunnel: [w1505 0 ("number")] -> w1451
              tunnel: [w1504 0] -> w1448
              tunnel: w1447 -> [w1503 w1803]
              tunnel: w1446 -> [w1502 _]
              tunnel: w1445 -> [w1501 _]
              tunnel: [w1500 w1803] -> w1444
              tunnel: [w1499 w1804] -> w1443
              tunnel: w1442 -> [w1498 _]
              tunnel: w1440 -> [w1490 _]
              tunnel: w1436 -> [w1470 _]
              tunnel: w1435 -> [w1469 _]
              frame #0 {
                n429 = flat-sequence {
                  tunnel: w1498 -> [w1516]
                  tunnel: w1506 -> [w1517]
                  tunnel: w1509 -> [w1518]
                  tunnel: w1510 -> [w1519]
                  tunnel: w1511 -> [w1520]
                  tunnel: w1512 -> [w1521]
                  tunnel: [w1521] -> w1489
                  tunnel: [w1520] -> w1487
                  tunnel: [w1519] -> w1485
                  tunnel: [w1518] -> w1483
                  tunnel: [w1517] -> w1481
                  tunnel: [w1516] -> w1479
                  tunnel: w1490 -> [w1514]
                  tunnel: w1489 -> [w1528]
                  tunnel: [w1528] -> w1488
                  tunnel: w1487 -> [w1527]
                  tunnel: [w1527] -> w1486
                  tunnel: w1485 -> [w1526]
                  tunnel: [w1526] -> w1484
                  tunnel: w1483 -> [w1525]
                  tunnel: [w1525] -> w1482
                  tunnel: w1481 -> [w1524]
                  tunnel: [w1524] -> w1480
                  tunnel: w1479 -> [w1523]
                  tunnel: [w1523] -> w1478
                  tunnel: [w1539] -> w1496
                  tunnel: [w1538] -> w1495
                  tunnel: [w1537] -> w1494
                  tunnel: [w1533] -> w1493
                  tunnel: [w1532] -> w1492
                  tunnel: [w1536] -> w1491
                  tunnel: w1488 -> [w1539]
                  tunnel: w1486 -> [w1538]
                  tunnel: w1484 -> [w1537]
                  tunnel: w1482 -> [w1535]
                  tunnel: w1480 -> [w1532]
                  tunnel: w1478 -> [w1536]
                  tunnel: [w1530] -> w1477
                  tunnel: w1468 -> [w1551]
                  tunnel: [w1550] -> w1505
                  tunnel: w1503 -> [w1547]
                  tunnel: w1502 -> [w1546]
                  tunnel: w1501 -> [w1545]
                  tunnel: w1496 -> [w1558]
                  tunnel: w1495 -> [w1557]
                  tunnel: w1494 -> [w1556]
                  tunnel: w1493 -> [w1555]
                  tunnel: w1492 -> [w1552]
                  tunnel: w1491 -> [w1542]
                  tunnel: w1477 -> [w1540]
                  tunnel: [w1554] -> w1467
                  tunnel: [w1553] -> w1466
                  tunnel: [w1549] -> w1465
                  tunnel: [w1548] -> w1464
                  tunnel: [w1544] -> w1463
                  tunnel: [w1543] -> w1462
                  tunnel: [w1793] -> w1499
                  tunnel: [w1794] -> w1500
                  tunnel: [w1795] -> w1504
                  tunnel: [w1796] -> w1507
                  tunnel: [w1797] -> w1508
                  tunnel: w1467 -> [w1797]
                  tunnel: w1466 -> [w1796]
                  tunnel: w1465 -> [w1766]
                  tunnel: w1464 -> [w1795]
                  tunnel: w1463 -> [w1794]
                  tunnel: w1462 -> [w1793]
                  frame #0 {
                    # "Go to N subsite"
                    n430 = Number To Decimal String(number=w1514) -> (decimal integer string=w1515:string)  [unwired: 1 in]
                    n431 = Wait (ms)(milliseconds to wait=u32 1500) -> ()  [unwired: 1 out]
                    n432 = call "-mov-prob-abs-subs.vi"("Subsite #"=w1515) -> ()  [unwired: 5 in]
                  }
                  frame #1 {
                    n433 = Wait (ms)(milliseconds to wait=u32 500) -> ()  [unwired: 1 out]
                  }
                  frame #2 {
                    n434 = local read "Bias Polarity"() -> (w1530:dbl)
                    n435 = call "Keith 237 Operate/Standby.vi"("source"=TRUE, "error in"=w1535, "GPIB address"=w1532) -> ("error out"=w1533:T2)
                    n436 = Wait (ms)(milliseconds to wait=u32 1000) -> ()  [unwired: 1 out]
                    n437 = local write "Status"("Starting CV Sensor Scan" ("Status")) -> ()
                  }
                  frame #3 {
                    w1541 = TRUE
                    n438 = while {
                      tunnel: w1552 -> [w1656]
                      tunnel: w1558 -> [w1583]
                      tunnel: w1557 -> [w1659]
                      tunnel: [w1641] -> w1553
                      tunnel: w1556 -> [w1642]
                      shift-right: [w1568] -> w1554
                      shift-left: w1555 -> [w1660]
                      tunnel: w1551 -> [w1654]
                      tunnel: [w1653] -> w1550
                      tunnel: [w1652] -> w1549
                      tunnel: [w1565] -> w1548
                      tunnel: w1547 -> [w1649]
                      tunnel: w1546 -> [w1647]
                      tunnel: w1545 -> [w1646]
                      tunnel: [w1645] -> w1544
                      tunnel: [w1630] -> w1543
                      tunnel: w1542 -> [w1588]
                      shift-right: [w1579] -> _
                      shift-left: w1541 -> [w1578]
                      shift-left: w1541 -> [w1562]
                      shift-left: w1541 -> [w1577]
                      shift-left: w1541 -> [w1561]
                      shift-left: w1541 -> [w1560]
                      tunnel: w1540 -> [w1559]
                      i -> [w1655]
                      stop <- w1572 continue-if-true
                      # "Only the K237 Bias and\nCapacitance are recorded in the \nXML file. The Excell file records \nK237 Bias, Capacitance, Secondary\nParameter, and Leakage Current\nas well as records the parameters\nset for the K237 and LCR meter"
                      # "Change Bias Polarity\n+1 Chuck Bias\n-1  Pad bias"
                      # "Plot Capacitance"
                      n439 = flat-sequence {
                        tunnel: w1642 -> [w1683]
                        tunnel: w1656 -> [w1684]
                        tunnel: w1660 -> [w1685]
                        tunnel: [w1685] -> w1617
                        tunnel: [w1684] -> w1616
                        tunnel: [w1683] -> w1615
                        tunnel: [w1682] -> w1595
                        tunnel: w1588 -> [w1681]
                        tunnel: w1653 -> [w1689]
                        tunnel: [w1690] -> w1614
                        tunnel: [w1688] -> w1612
                        tunnel: [w1687] -> w1610
                        tunnel: w1617 -> [w1691]
                        tunnel: w1616 -> [w1687]
                        tunnel: w1615 -> [w1688]
                        tunnel: [w1686] -> w1596
                        tunnel: w1595 -> [w1686]
                        tunnel: w1614 -> [w1696]
                        tunnel: [w1696] -> w1613
                        tunnel: w1612 -> [w1695]
                        tunnel: [w1695] -> w1611
                        tunnel: w1610 -> [w1694]
                        tunnel: [w1694] -> w1609
                        tunnel: w1596 -> [w1693]
                        tunnel: [w1692] -> w1593
                        tunnel: w1613 -> [w1701]
                        tunnel: [w1700] -> w1608
                        tunnel: [w1699] -> w1606
                        tunnel: w1611 -> [w1699]
                        tunnel: [w1698] -> w1604
                        tunnel: w1609 -> [w1698]
                        tunnel: [w1697] -> w1594
                        tunnel: w1593 -> [w1697]
                        tunnel: w1608 -> [w1706]
                        tunnel: [w1706] -> w1607
                        tunnel: w1606 -> [w1705]
                        tunnel: [w1705] -> w1605
                        tunnel: w1604 -> [w1704]
                        tunnel: [w1704] -> w1603
                        tunnel: w1594 -> [w1703]
                        tunnel: [w1702] -> w1589
                        tunnel: w1607 -> [w1709]
                        tunnel: w1605 -> [w1712]
                        tunnel: [w1708] -> w1629
                        tunnel: [w1712] -> w1628
                        tunnel: [w1711] -> w1627
                        tunnel: [w1710] -> w1626
                        tunnel: w1603 -> [w1710]
                        tunnel: [w1707] -> w1590
                        tunnel: w1589 -> [w1707]
                        tunnel: w1629 -> [w1724]
                        tunnel: [w1724] -> w1625
                        tunnel: w1628 -> [w1723]
                        tunnel: [w1723] -> w1624
                        tunnel: w1627 -> [w1722]
                        tunnel: [w1722] -> w1623
                        tunnel: w1626 -> [w1721]
                        tunnel: [w1721] -> w1622
                        tunnel: [w1719] -> w1591
                        tunnel: w1590 -> [w1719]
                        tunnel: w1625 -> [w1733]
                        tunnel: [w1733] -> w1602
                        tunnel: w1624 -> [w1732]
                        tunnel: [w1732] -> w1600
                        tunnel: w1623 -> [w1731]
                        tunnel: [w1731] -> w1598
                        tunnel: w1622 -> [w1726]
                        tunnel: [w1728] -> w1620
                        tunnel: [w1727] -> w1592
                        tunnel: w1591 -> [w1727]
                        tunnel: [w1726] -> w1584
                        tunnel: [w1725] -> w1580
                        tunnel: w1602 -> [w1738]
                        tunnel: [w1738] -> w1601
                        tunnel: w1600 -> [w1737]
                        tunnel: [w1737] -> w1599
                        tunnel: w1598 -> [w1736]
                        tunnel: [w1736] -> w1597
                        tunnel: w1592 -> [w1735]
                        tunnel: [w1734] -> w1585
                        tunnel: w1584 -> [w1734]
                        tunnel: w1601 -> [w1746]
                        tunnel: w1599 -> [w1745]
                        tunnel: w1597 -> [w1741]
                        tunnel: [w1746] -> w1640
                        tunnel: [w1745] -> w1639
                        tunnel: [w1741] -> w1638
                        tunnel: w1585 -> [w1739]
                        tunnel: [w1739] -> w1581
                        tunnel: w1640 -> [w1753]
                        tunnel: w1639 -> [w1752]
                        tunnel: w1638 -> [w1748]
                        tunnel: [w1753] -> w1637
                        tunnel: [w1752] -> w1636
                        tunnel: [w1748] -> w1635
                        tunnel: w1637 -> [w1760]
                        tunnel: w1636 -> [w1759]
                        tunnel: w1635 -> [w1758]
                        tunnel: [w1760] -> w1634
                        tunnel: [w1759] -> w1633
                        tunnel: [w1756] -> w1632
                        tunnel: [w1754] -> w1621
                        tunnel: [w1763] -> w1567
                        tunnel: [w1764] -> w1641
                        tunnel: [w1765] -> w1631
                        tunnel: w1634 -> [w1765]
                        tunnel: w1633 -> [w1764]
                        tunnel: w1632 -> [w1763]
                        tunnel: [w1761] -> w1571
                        tunnel: w1621 -> [w1761]
                        frame #0 {
                          n440 = call <vilib>:"Acquire Semaphore.vi"("semaphore"=w1681) -> ("semaphore out"=w1682:T1)  [unwired: 4 in, 2 out]
                        }
                        frame #1 {
                          # "Set Voltage"
                          n441 = call "Kei237_Set_Volt.vi"("Voltage"=w1689, "error in"=w1691, "GPIB"=w1687) -> ("error out"=w1690:errorcluster)
                        }
                        frame #2 {
                          n442 = call <vilib>:"Release Semaphore.vi"("semaphore"=w1693) -> ("semaphore out"=w1692:T1)  [unwired: 5 in, 1 out]
                        }
                        frame #3 {
                          n443 = call "Time Delay3"("error in (no error)"=w1701) -> ("error out"=w1700:errorcluster)  [unwired: 10 in]
                        }
                        frame #4 {
                          n444 = call <vilib>:"Acquire Semaphore.vi"("semaphore"=w1703) -> ("semaphore out"=w1702:T1)  [unwired: 4 in, 2 out]
                        }
                        frame #5 {
                          n445 = call "7000 Series Aquire Data.vi"("inst handle in"=w1712, "error in"=w1709) -> ("Primary"=w1713:string, "Primary Value"=w1714:string, "Primary Unit"=w1715:string, "Secondary"=w1718:string, "Secondary Value"=w1717:string, "Secondary Unit"=w1716:string, "error out"=w1708:T8)  [unwired: 5 in, 2 out]
                          n446 = Bundle("Primary"=w1713, "Primary Value"=w1714, "Primary Unit"=w1715, "Secondary"=w1718, "Secondary Value"=w1717, "Secondary Unit"=w1716) -> (w1711:T10)  [unwired: 1 in]
                        }
                        frame #6 {
                          n447 = Wait (ms)(milliseconds to wait=200) -> ()  [unwired: 1 out]
                        }
                        frame #7 {
                          n448 = call "K237-read-current-2.vi"("GPIB"=w1726) -> ("Current"=w1728:dbl)  [unwired: 1 in, 1 out]
                          "Total Current" <- w1728
                          n449 = local read "Compliance"() -> (w1729:dbl)
                          n450 = Absolute Value(x=w1728) -> (abs(x)=w1730:dbl)
                          n451 = Greater Or Equal?(x=w1730, y=w1729) -> (x >= y?=w1725:bool)
                          "Compliance" <- w1725
                        }
                        frame #8 {
                          n452 = call <vilib>:"Release Semaphore.vi"("semaphore"=w1735) -> ()  [unwired: 5 in, 2 out]
                        }
                        frame #9 {
                          n453 = Unbundle(w1741) -> ("Primary"=w1742:string, "Primary Unit"=w1743:string)  [unwired: 4 out]
                          n454 = call <vilib>:"Space Constant.vi"() -> ("String"=w1740:string)
                          n455 = Concatenate Strings(w1742, w1740, w1743) -> (w1744:string)
                          n456 = property on="Capacitance" class="XYGraph (strict)"("Caption.Text"=w1742, "YScale.NameLbl.Text"=w1744) -> ()  [unwired: 2 in, 2 out]
                        }
                        frame #10 {
                          n457 = call <vilib>:"Space Constant.vi"() -> ("String"=w1747:string)
                          n458 = Unbundle(w1748) -> ("Secondary"=w1750:string, "Secondary Unit"=w1749:string)  [unwired: 4 out]
                          n459 = Concatenate Strings(w1750, w1747, w1749) -> (w1751:string)
                          n460 = property on="Secondary Parameter Graph" class="XYGraph (strict)"("Caption.Text"=w1750, "YScale.NameLbl.Text"=w1751) -> ()  [unwired: 2 in, 2 out]
                        }
                        frame #11 {
                          n461 = Unbundle(w1758) -> ("Primary Value"=w1757:string, "Secondary Value"=w1755:string)  [unwired: 4 out]
                          n462 = Fract/Exp String To Number(string=w1757) -> (number=w1756:dbl)  [unwired: 3 in, 1 out]
                          n463 = Fract/Exp String To Number(string=w1755) -> (number=w1754:dbl)  [unwired: 3 in, 1 out]
                        }
                        frame #12 {
                          n464 = Wait (ms)(milliseconds to wait=200) -> ()  [unwired: 1 out]
                        }
                      }
                      n465 = Build Array(w1578, w1577, w1562, w1561, w1560) -> (w1576:bool[])
                      n466 = Multiply(x=w1659, y=w1655) -> (x*y=w1565:i32)
                      n467 = local write "K237_Bias"(w1565) -> ()
                      n468 = Multiply(x=w1559, y=w1565) -> (x*y=w1653:dbl)
                      n469 = Or Array Elements(Boolean array=w1576) -> (logical OR=w1573:bool)
                      n470 = Equal To 0?(x=w1655) -> (x = 0?=w1570:bool)
                      n471 = case shown="True" "Halt CV" {
                        selector: "Halt CV" -> [_ w1668]
                        tunnel: [FALSE ("source") w1669] -> w1651
                        tunnel: w1581 -> [_ w1664]
                        frame #0 {
                        }
                        frame #1 {
                          n472 = flat-sequence {
                            tunnel: w1668 -> [w1672]
                            tunnel: [w1672] -> w1667
                            tunnel: w1664 -> [w1670]
                            tunnel: [w1670] -> w1662
                            tunnel: w1667 -> [w1674]
                            tunnel: [w1675] -> w1666
                            tunnel: [w1673] -> w1663
                            tunnel: w1662 -> [w1673]
                            tunnel: w1666 -> [w1678]
                            tunnel: [w1678] -> w1665
                            tunnel: w1663 -> [w1676]
                            tunnel: [w1680] -> w1669
                            tunnel: w1665 -> [w1680]
                            frame #0 {
                              n473 = call "Keith 237 Operate/Standby.vi"("source"=FALSE, "GPIB address"=w1670) -> ()  [unwired: 1 in, 1 out]
                            }
                            frame #1 {
                              n474 = call "Prompt User for Input2"("Enable"=w1674) -> ("Yes"=w1675:bool)  [unwired: 17 in, 1 out]
                            }
                            frame #2 {
                              n475 = call "Keith 237 Operate/Standby.vi"("source"=TRUE, "GPIB address"=w1676) -> ()  [unwired: 1 in, 1 out]
                            }
                            frame #3 {
                              n476 = Wait (ms)(milliseconds to wait=750) -> ()  [unwired: 1 out]
                            }
                          }
                        }
                      }
                      n477 = Not(x=w1580) -> (.not. x?=w1579:bool)
                      n478 = Absolute Value(x=w1565) -> (abs(x)=w1644:i32)
                      n479 = Absolute Value(x=w1583) -> (abs(x)=w1643:i32)
                      n480 = Less?(x=w1644, y=w1643) -> (x < y?=w1574:bool)
                      n481 = Not(x=w1651) -> (.not. x?=w1575:bool)
                      n482 = Compound Arithmetic op=AND(w1573, w1574, w1575) -> (w1572:bool)
                      n483 = call "Primary"("error in (no error)"=w1631, "Reset"=w1570, "Y Input"=w1567, "X Input"=w1565) -> ("error out"=w1618:errorcluster, "XY Graph"=w1587:cluster{"Y":dbl[], "Y":dbl[]}[])  [unwired: 1 in, 5 out]
                      n484 = call "Secondary"("error in (no error)"=w1618, "Reset"=w1570, "Y Input"=w1571, "X Input"=w1565) -> ("error out"=w1569:errorcluster, "XY Graph"=w1586:cluster{"Y":dbl[], "Y":dbl[]}[])  [unwired: 1 in, 5 out]
                      n485 = Square(x=w1567) -> (x^2=w1566:dbl)
                      n486 = Reciprocal(x=w1566) -> (1/x=w1564:dbl)
                      n487 = call "1/C^2"("error in (no error)"=w1569, "Reset"=w1570, "Y Input"=w1564, "X Input"=w1565) -> ("error out"=w1568:errorcluster, "XY Graph"=w1563:cluster{"Y":dbl[], "Y":dbl[]}[])  [unwired: 1 in, 5 out]
                      n488 = local write "Secondary Parameter Graph"(w1586) -> ()
                      n489 = local write "1/C^2"(w1563) -> ()
                      n490 = Build Array(w1565, w1567) -> (w1650:dbl[])
                      n491 = Build Array(w1565, w1567, w1571, w1620, w1564) -> (w1619:dbl[])
                      n492 = call "XML_Data.vi"("Data Input Array"=w1650, "Data Tag Names Array"=w1646, "XML File Path"=w1647, "DOM document in"=w1649) -> ("DOM document out"=w1645:refnum<k20>)  [unwired: 6 in, 1 out]
                      n493 = call-poly <vilib>:"Write To Spreadsheet File.vi"("delimiter (\\t)"="," ("delimiter (\\t)"), "format (%.3f)"="%.3e" ("file format"), "append to file? (new file:F)"=TRUE, "1D data"=w1619, "file path (dialog if empty)"=w1654) -> ("new file path (Not A Path if cancelled)"=w1652:path)  [unwired: 2 in, 1 out]
                      n494 = local write "Capacitance"(w1587) -> ()
                      n495 = Bundle("XY Graph"=w1587, "XY Graph"=w1586, "XY Graph"=w1563) -> (w1630:T11)  [unwired: 1 in]
                    }
                  }
                  frame #4 {
                    # "The Parameters that are appended\nto the Excell file"
                    n496 = local read "Frequency"() -> (w1792:dbl)
                    n497 = local read "Voltage Level"() -> (w1791:dbl)
                    n498 = local read "CV-V-Steps"() -> (w1785:i32)
                    n499 = local read "Number of Averages"() -> (w1784:dbl)
                    n500 = local read "Time Delay mS"() -> (w1783:dbl)
                    n501 = local read "Voltage Range"() -> (w1780:string)
                    n502 = property on="Primary Parameter" class="Ring (strict)"() -> ("RingText.Text"=w1779:string)  [unwired: 2 in, 2 out]
                    n503 = property on="Secondary Parameter" class="Ring (strict)"() -> ("RingText.Text"=w1767:string)  [unwired: 2 in, 2 out]
                    n504 = Number To Exponential String(number=w1792) -> (E-format string=w1789:string)  [unwired: 3 in]
                    n505 = Number To Exponential String(number=w1791) -> (E-format string=w1788:string)  [unwired: 3 in]
                    n506 = Number To Exponential String(number=w1785) -> (E-format string=w1787:string)  [unwired: 3 in]
                    n507 = Number To Exponential String(number=w1784) -> (E-format string=w1786:string)  [unwired: 3 in]
                    n508 = Number To Exponential String(number=w1783) -> (E-format string=w1781:string)  [unwired: 3 in]
                    n509 = Build Array("LCR Parameters" ("element"), "Frequency", "Voltage Level", "Voltage Step", "Number of Averages", "Time Delay mS", "Voltage Range (K237)", "Primary", "Secondary") -> (w1771:string[])
                    n510 = Build Array("", w1789, w1788, w1787, w1786, w1781, w1780, w1779, w1767) -> (w1770:string[])
                    n511 = Build Array(w1771, w1770) -> (w1769:string[][])
                    n512 = call "Manual CV paramter_append.vi"("Array"=w1769, "Path"=w1766) -> ()  [unwired: 9 in, 1 out]
                  }
                }
                n513 = local write "Running Conditional"(TRUE) -> ()
                n514 = Open/Create/Replace File(file path (use dialog)=w1470, operation (0:open)=T5."replace or create", access (0:read/write)=enum16{"read/write", "read-only", "write-only"}."read/write") -> (refnum out=w1473:refnum<file>)  [unwired: 1 in, 4 out]
                n515 = Refnum to Path(1:w1473) -> (0:w1474:path)
                n516 = call-poly <vilib>:"Write To Spreadsheet File.vi"("delimiter (\\t)"="," ("delimiter (\\t)"), "append to file? (new file:F)"=FALSE, "2D data"=w1469, "file path (dialog if empty)"=w1474) -> ("new file path (Not A Path if cancelled)"=w1468:path)  [unwired: 4 in]
              }
              frame #1 {
                w1798 = cluster{"Y":dbl[], "Y":dbl[]}[] [] ("XY Graph")
                n517 = Bundle("XY Graph"=w1798, "XY Graph"=w1798, "XY Graph"=w1798) -> (w1804:T11)  [unwired: 1 in]
              }
            }
            n518 = Number To Fractional String(number=0) -> (F-format string=w1452:string)  [unwired: 3 in]
            n519 = Number To Fractional String(number=w1451) -> (F-format string=w1453:string)  [unwired: 3 in]
            n520 = Concatenate Strings(w1452, " : ", w1453) -> (→"Voltage Range":string)
            n521 = call-poly <vilib>:"Close.vi"("node"=w1444) -> ()  [unwired: 8 in, 1 out]
          }
          frame #2 {
            w1805 = FALSE
            n522 = local write "Running Conditional"(w1805) -> ()
            n523 = local write "Running?"(w1805) -> ()
          }
          frame #3 {
            n524 = case shown="True" FALSE {
              tunnel: w1817 -> [w1820 w1825]
              tunnel: [w1820 w1824] -> w1816
              tunnel: w1815 -> [w1819 w1823]
              tunnel: [w1819 w1822] -> w1814
              tunnel: w1813 -> [_ w1821]
              frame #0 {
              }
              frame #1 {
                n525 = while {
                  tunnel: [w1841] -> w1822
                  tunnel: w1823 -> [w1835]
                  tunnel: w1825 -> [w1834]
                  tunnel: [w1834] -> w1824
                  tunnel: w1821 -> [w1828]
                  i -> [w1840]
                  stop <- w1837 continue-if-true
                  n526 = Multiply(x=25, y=w1840) -> (x*y=w1831:i32)
                  n527 = Sign(1:w1828) -> (0:w1833:i32)
                  n528 = Subtract(x=w1828, y=w1831) -> (x-y=w1830:i32)
                  n529 = Add(x=w1828, y=w1831) -> (x+y=w1829:i32)
                  n530 = Greater Than 0?(x=w1833) -> (x > 0?=w1832:bool)
                  n531 = Select(t=w1830, s=w1832, f=w1829) -> (s? t:f=w1826:i32)
                  n532 = Absolute Value(x=w1826) -> (abs(x)=w1827:i32)
                  n533 = local write "K237_Bias"(w1826) -> ()
                  n534 = call "Time Delay2"("error in (no error)"=w1835) -> ("error out"=w1836:errorcluster)  [unwired: 10 in]
                  n535 = Greater?(x=w1827, y=25) -> (0:w1837:bool)
                  n536 = call "Kei237_Set_Volt.vi"("Voltage"=w1826, "error in"=w1836, "GPIB"=w1834) -> ("error out"=w1841:errorcluster)
                }
              }
            }
          }
          frame #4 {
            n537 = Wait (ms)(milliseconds to wait=250) -> ()  [unwired: 1 out]
          }
          frame #5 {
            w1858 = 0
            n538 = In Range and Coerce(upper limit=3, x=w1852, lower limit=0) -> (In Range?=w1863:bool)  [unwired: 1 out]
            n539 = property on="Archive" class="TabCtl (strict)"("Value"=4) -> ()  [unwired: 2 in, 2 out]
            n540 = call "Kei237_Set_Volt.vi"("Voltage"=w1858, "error in"=w1868, "GPIB"=w1850) -> ("error out"=w1851:errorcluster)
            n541 = Wait Until Next ms Multiple(millisecond multiple=u32 250) -> ()  [unwired: 1 out]
            n542 = case shown="False" w1863 {
              tunnel: [w1890 0] -> w1862
              tunnel: w1852 -> [w1888 _]
              frame #0 {
                n543 = In Range and Coerce(upper limit=11, x=w1888, lower limit=4) -> (In Range?=w1889:bool)  [unwired: 1 out]
                n544 = case shown="False" w1889 {
                  tunnel: [2 1] -> w1890
                  frame #0 {
                  }
                  frame #1 {
                  }
                }
              }
              frame #1 {
              }
            }
            n545 = call "Keith 237 Operate/Standby.vi"("source"=FALSE, "error in"=w1851, "GPIB address"=w1850) -> ("error out"=w1848:T2)
            n546 = local write "K237_Bias"(w1858) -> ()
            n547 = Unbundle(w1856) -> (w1855:cluster{"Y":dbl[], "Y":dbl[]}[], w1854:cluster{"Y":dbl[], "Y":dbl[]}[], w1853:cluster{"Y":dbl[], "Y":dbl[]}[])
            n548 = local write "Status"("Finshing CV Sensor Scan" ("Status")) -> ()
            n549 = case shown="0, Default" w1862 {
              tunnel: [w1875 w1881 w1887] -> w1861
              tunnel: w1855 -> [w1874 w1881 w1887]
              tunnel: [w1873 w1880 w1886] -> w1860
              tunnel: w1854 -> [w1873 w1879 w1886]
              tunnel: [w1872 w1878 w1885] -> w1859
              tunnel: w1853 -> [w1872 w1878 w1884]
              tunnel: w1857 -> [w1871 w1877 w1883]
              frame #0 {
                # "Diodes"
                n550 = Unbundle(w1871) -> ("XY Graph"=w1870:cluster{"Y":dbl[], "Y":dbl[]}[])  [unwired: 2 out]
                n551 = Insert Into Array(array=w1874, new element=w1870) -> (w1875:cluster{"Y":dbl[], "Y":dbl[]}[])  [unwired: 1 in]
                "Diodes Capacitance" <- w1875
              }
              frame #1 {
                # "2x8s"
                n552 = Unbundle(w1877) -> ("XY Graph"=w1876:cluster{"Y":dbl[], "Y":dbl[]}[])  [unwired: 2 out]
                n553 = Insert Into Array(array=w1879, new element=w1876) -> (w1880:cluster{"Y":dbl[], "Y":dbl[]}[])  [unwired: 1 in]
                "2x8 Chip Capacitance" <- w1880
              }
              frame #2 {
                # "Single Chips"
                n554 = Unbundle(w1883) -> ("XY Graph"=w1882:cluster{"Y":dbl[], "Y":dbl[]}[])  [unwired: 2 out]
                n555 = Insert Into Array(array=w1884, new element=w1882) -> (w1885:cluster{"Y":dbl[], "Y":dbl[]}[])  [unwired: 1 in]
                "Single Chip Capacitance" <- w1885
              }
            }
          }
        }
        n556 = Concatenate Strings(w1342, "_CV.csv" ("string")) -> (w1383:string)
        n557 = Concatenate Strings(w1342, "_CV.xml" ("string")) -> (w1381:string)
        n558 = property on="Primary Parameter" class="Ring (strict)"() -> ("RingText.Text"=w1373:string)  [unwired: 2 in, 2 out]
        n559 = property on="Secondary Parameter" class="Ring (strict)"() -> ("RingText.Text"=w1370:string)  [unwired: 2 in, 2 out]
        n560 = Build Path(base path=w1380, name or relative path=w1383) -> (appended path=w1340:path)
        n561 = Build Array("Bias", w1373, w1370, "Leakage Current" ("element"), "1/C^2" ("element")) -> (w1397:string[])
        n562 = Build Path(base path=w1338, name or relative path=w1381) -> (appended path=w1379:path)
        n563 = Build Array(w1341, w1397) -> (w1339:string[][])
        n564 = Build Array("VOLTAGE_VOLT", "ACTV_CAP_FRD") -> (w1376:string[])
        n565 = call "XML_Initilize.vi"("User Input"=w1343) -> ("DOM document out"=w1385:refnum<k20>)  [unwired: 10 in]
      }
      n566 = call "7000 Series Configure.vi"("inst handle in"=w1332, "error in"=w1331, "Bias"=w1334) -> ("inst handle out"=w1333:refnum<visa-resource-name>, "error out"=w1329:T8)  [unwired: 22 in, 1 out]
      n567 = call "Keith 237 Reset.vi"("GPIB address"=w1330, "error in"=w1329) -> ("error out"=w1328:T2)
      n568 = call "7000 Series Close.vi"("error in (no error)"=w1328, "VISA session"=w1333) -> ("error out"=w1325:errorcluster)
    }
    frame #8 {
      n569 = local write "Stop Loop"(w1897) -> ()
      n570 = local write "Status"("Finished Full CV Scan" ("Status")) -> ()
      n571 = Wait (ms)(milliseconds to wait=u32 500) -> ()  [unwired: 1 out]
    }
    frame #9 {
      n572 = Build Array(16) -> (w1904:i32[])
      n573 = local write "Stop Loop"(TRUE ("Stop Loop")) -> ()
      n574 = EnableLocal(2:w1903, 3:w1904, 4:0) -> (0:→"error out":errorcluster)  [unwired: 1 out]
      n575 = local write "Status"("Full Automatic Scan Completed" ("Status")) -> ()
    }
  }
  n576 = call <vilib>:"Check if File or Folder Exists.vi"("path"=w25) -> ("file or folder exists?"=w24:bool, "dup path"=w23:path)  [unwired: 8 in, 1 out]
  n577 = case shown="False" w24 {
    tunnel: w23 -> [w1911 w1912]
    tunnel: [w1910 w1912] -> w2
    frame #0 {
      n578 = Create Folder(path (use dialog)=w1911) -> (created path=w1910:path)  [unwired: 2 in, 2 out]
    }
    frame #1 {
    }
  }
  n579 = while {
    tunnel: [w1914] -> _
    tunnel: w35 -> [w1914]
    stop <- "Stop Loop" continue-if-true
    n580 = call <vilib>:"Acquire Semaphore.vi"("semaphore"=w1914) -> ("semaphore out"=w1917:T1)  [unwired: 4 in, 2 out]
    n581 = Wait (ms)(milliseconds to wait=50) -> ()  [unwired: 1 out]
    n582 = case shown="True" "Emergency Stop" {
      selector: "Emergency Stop" -> [_ w1924]
      tunnel: w1917 -> [w1920 w1923]
      tunnel: [w1920 w1923] -> w1916
      tunnel: "IV or CV" -> [_ w1922]
      frame #0 {
      }
      frame #1 {
        n583 = case shown="0, Default" w1922 {
          tunnel: w1924 -> [w1926 w1986]
          tunnel: w1923 -> [w1925 w1985]
          frame #0 {
            n584 = flat-sequence {
              tunnel: [w1937] -> w1929
              tunnel: w1926 -> [w1937]
              tunnel: w1925 -> [w1934]
              tunnel: [w1934] -> w1928
              tunnel: w1929 -> [w1983]
              tunnel: [w1983] -> w1927
              tunnel: w1928 -> [w1982]
              tunnel: w1927 -> [w1984]
              frame #0 {
                n585 = flat-sequence {
                  tunnel: [w1938] -> w1935
                  tunnel: w1935 -> [w1944]
                  tunnel: [w1945] -> w1933
                  tunnel: [w1946] -> w1931
                  tunnel: w1933 -> [w1967]
                  tunnel: [w1967] -> w1932
                  tunnel: w1931 -> [w1966]
                  tunnel: [w1966] -> w1930
                  tunnel: [w1971] -> w1936
                  tunnel: w1932 -> [w1969]
                  tunnel: w1930 -> [w1968]
                  tunnel: w1936 -> [w1978]
                  frame #0 {
                    n586 = call "KE6485 Close.vi"("instrument handle"=refnum<k15> "GPIB0::10::INSTR") -> ("error out"=w1941:errorcluster)  [unwired: 10 in]
                    n587 = Wait (ms)(milliseconds to wait=2000) -> ()  [unwired: 1 out]
                    n588 = call "KE6485 Close.vi"("error in (no error)"=w1941, "instrument handle"=refnum<k15> "GPIB0::14::INSTR") -> ("error out"=w1938:errorcluster)  [unwired: 9 in]
                  }
                  frame #1 {
                    n589 = local read "K237_Bias"() -> (w1943:dbl)
                    n590 = while {
                      tunnel: [w1964] -> w1945
                      tunnel: "16" ("GPIB") -> [w1960]
                      tunnel: [w1960] -> w1946
                      shift-right: [w1949] -> _
                      shift-left: w1943 -> [w1955]
                      tunnel: w1944 -> [w1948]
                      i -> [w1951]
                      stop <- w1952 continue-if-true
                      n591 = Sign(1:w1955) -> (0:w1953:dbl)
                      n592 = Sign(1:w1951) -> (0:w1950:i32)
                      n593 = Greater Than 0?(x=w1953) -> (x > 0?=w1959:bool)
                      n594 = Multiply(x=25, y=w1950) -> (x*y=w1958:i32)
                      n595 = Subtract(x=w1955, y=w1958) -> (x-y=w1957:dbl)
                      n596 = Add(x=w1955, y=w1958) -> (x+y=w1956:dbl)
                      n597 = Select(t=w1957, s=w1959, f=w1956) -> (s? t:f=w1949:dbl)
                      n598 = Absolute Value(x=w1949) -> (abs(x)=w1954:dbl)
                      n599 = call "Time Delay5"("error in (no error)"=w1948) -> ("error out"=w1961:errorcluster)  [unwired: 10 in]
                      n600 = Greater?(x=w1954, y=25) -> (0:w1952:bool)
                      n601 = call "Kei237_Set_Volt.vi"("Voltage"=w1949, "error in"=w1961, "GPIB"=w1960) -> ("error out"=w1964:errorcluster)
                    }
                  }
                  frame #2 {
                    n602 = Wait (ms)(milliseconds to wait=750) -> ()  [unwired: 1 out]
                  }
                  frame #3 {
                    n603 = call "Kei237_Set_Volt.vi"("Voltage"=0, "error in"=w1969, "GPIB"=w1968) -> ("error out"=w1973:errorcluster)
                    n604 = call "Keith 237 Reset.vi"("GPIB address"=w1968, "error in"=w1973) -> ("error out"=w1971:T2)
                    n605 = Wait (ms)(milliseconds to wait=750) -> ()  [unwired: 1 out]
                  }
                  frame #4 {
                    n606 = Build Array(16, 10, 14) -> (w1974:i32[])
                    n607 = EnableLocal(2:w1978, 3:w1974, 4:0) -> (0:→"error out 6":errorcluster)  [unwired: 1 out]
                  }
                }
              }
              frame #1 {
                w1981 = FALSE ("Emergency Stop")
                n608 = local write "Emergency Stop"(w1981) -> ()
                n609 = local write "Bias Loop"(w1981) -> ()
                n610 = call <vilib>:"Release Semaphore Reference.vi"("semaphore"=w1982) -> ()  [unwired: 9 in, 2 out]
              }
              frame #2 {
                n611 = Stop(stop? (T)=w1984) -> ()
              }
            }
          }
          frame #1 {
            n612 = flat-sequence {
              tunnel: [w1997] -> w1989
              tunnel: w1986 -> [w1997]
              tunnel: w1985 -> [w1995]
              tunnel: [w1995] -> w1988
              tunnel: w1989 -> [w2042]
              tunnel: [w2042] -> w1987
              tunnel: w1988 -> [w2041]
              tunnel: w1987 -> [w2043]
              frame #0 {
                n613 = flat-sequence {
                  tunnel: [w2001] -> w1994
                  tunnel: [w2006] -> w1993
                  tunnel: [w2007] -> w1991
                  tunnel: w1994 -> [w2004]
                  tunnel: w1993 -> [w2028]
                  tunnel: [w2028] -> w1992
                  tunnel: w1991 -> [w2027]
                  tunnel: [w2027] -> w1990
                  tunnel: [w2032] -> w1996
                  tunnel: w1992 -> [w2029]
                  tunnel: w1990 -> [w2030]
                  tunnel: w1996 -> [w2037]
                  frame #0 {
                    w1999 = u16 0 items=["Off", "Internal", "External"] ("Bias")
                    n614 = call "7000 Series Configure.vi"("inst handle in"=refnum<visa-resource-name> "GPIB0::4::INSTR", "Bias"=w1999) -> ("inst handle out"=w2003:refnum<visa-resource-name>, "error out"=w2002:T8)  [unwired: 23 in, 1 out]
                    n615 = Wait (ms)(milliseconds to wait=2000) -> ()  [unwired: 1 out]
                    n616 = call "7000 Series Close.vi"("error in (no error)"=w2002, "VISA session"=w2003) -> ("error out"=w2001:errorcluster)
                  }
                  frame #1 {
                    n617 = local read "K237_Bias"() -> (w2005:dbl)
                    n618 = while {
                      tunnel: [w2025] -> w2006
                      tunnel: "16" ("GPIB") -> [w2021]
                      tunnel: [w2021] -> w2007
                      shift-right: [w2010] -> _
                      shift-left: w2005 -> [w2016]
                      tunnel: w2004 -> [w2009]
                      i -> [w2012]
                      stop <- w2013 continue-if-true
                      n619 = Sign(1:w2016) -> (0:w2014:dbl)
                      n620 = Sign(1:w2012) -> (0:w2011:i32)
                      n621 = Greater Than 0?(x=w2014) -> (x > 0?=w2020:bool)
                      n622 = Multiply(x=25, y=w2011) -> (x*y=w2019:i32)
                      n623 = Subtract(x=w2016, y=w2019) -> (x-y=w2018:dbl)
                      n624 = Add(x=w2016, y=w2019) -> (x+y=w2017:dbl)
                      n625 = Select(t=w2018, s=w2020, f=w2017) -> (s? t:f=w2010:dbl)
                      n626 = Absolute Value(x=w2010) -> (abs(x)=w2015:dbl)
                      n627 = call "Time Delay6"("error in (no error)"=w2009) -> ("error out"=w2022:errorcluster)  [unwired: 10 in]
                      n628 = Greater?(x=w2015, y=25) -> (0:w2013:bool)
                      n629 = call "Kei237_Set_Volt.vi"("Voltage"=w2010, "error in"=w2022, "GPIB"=w2021) -> ("error out"=w2025:errorcluster)
                    }
                  }
                  frame #2 {
                    n630 = Wait (ms)(milliseconds to wait=750) -> ()  [unwired: 1 out]
                  }
                  frame #3 {
                    n631 = call "Kei237_Set_Volt.vi"("Voltage"=0, "error in"=w2029, "GPIB"=w2030) -> ("error out"=w2034:errorcluster)
                    n632 = Wait (ms)(milliseconds to wait=750) -> ()  [unwired: 1 out]
                    n633 = call "Keith 237 Reset.vi"("GPIB address"=w2030, "error in"=w2034) -> ("error out"=w2032:T2)
                  }
                  frame #4 {
                    n634 = Build Array(16) -> (w2035:i32[])
                    n635 = EnableLocal(2:w2037, 3:w2035, 4:0) -> (0:→"error out 7":errorcluster)  [unwired: 1 out]
                  }
                }
              }
              frame #1 {
                w2040 = FALSE ("Emergency Stop")
                n636 = local write "Emergency Stop"(w2040) -> ()
                n637 = local write "Bias Loop"(w2040) -> ()
                n638 = call <vilib>:"Release Semaphore Reference.vi"("semaphore"=w2041) -> ()  [unwired: 9 in, 2 out]
              }
              frame #2 {
                n639 = Stop(stop? (T)=w2043) -> ()
              }
            }
          }
        }
        n640 = local write "Status"("Emergency Stop" ("Status")) -> ()
      }
    }
    n641 = call <vilib>:"Release Semaphore.vi"("semaphore"=w1916) -> ()  [unwired: 5 in, 2 out]
  }
  n642 = List Folder(path=w2) -> (path out=w7:path, folder names=w4:string[])  [unwired: 3 in, 2 out]
  n643 = for {
    tunnel: w4 -> [w2046] mode=indexing
    shift-right: [w2045] -> w6
    shift-left: w3 -> [w2044]
    n644 = Equal?(x=w2044, y=w2046) -> (x = y?=w2047:bool)
    n645 = case shown="True" w2047 {
      tunnel: w2044 -> [_ w2056]
      tunnel: [w2048 w2049] -> w2045
      tunnel: w2044 -> [w2048 _]
      frame #0 {
      }
      frame #1 {
        n646 = Concatenate Strings("_(", "[0-9]+" ("string"), ")" ("string")) -> (w2063:string)
        n647 = Match Pattern(string=w2056, regular expression=w2063) -> (before substring=w2051:string, match substring=w2055:string)  [unwired: 1 in, 2 out]
        n648 = Match Pattern(string=w2055, regular expression="[0-9]+" ("string")) -> (match substring=w2062:string)  [unwired: 1 in, 3 out]
        n649 = Decimal String To Number(string=w2062) -> (number=w2061:i32)  [unwired: 2 in, 1 out]
        n650 = Increment(x=w2061) -> (x+1=w2060:i32)
        n651 = Number To Decimal String(number=w2060) -> (decimal integer string=w2059:string)  [unwired: 1 in]
        n652 = Concatenate Strings("_(", w2059, ")") -> (w2052:string)
        n653 = Concatenate Strings(w2051, w2052) -> (w2049:string)
      }
    }
  }
  n654 = Build Path(base path=w7, name or relative path=w6) -> (appended path=w5:path)
  n655 = Create Folder(path (use dialog)=w5) -> (created path=w1:path)  [unwired: 2 in, 2 out]
  n656 = Build Path(base path=w1, name or relative path="XML") -> (appended path=w9:path)
  n657 = call <vilib>:"Check if File or Folder Exists.vi"("path"=w9) -> ("file or folder exists?"=w12:bool, "dup path"=w11:path)  [unwired: 8 in, 1 out]
  n658 = case shown="False" w12 {
    tunnel: w11 -> [w2066 w2067]
    tunnel: [w2065 w2067] -> w8
    frame #0 {
      n659 = Create Folder(path (use dialog)=w2066) -> (created path=w2065:path)  [unwired: 2 in, 2 out]
    }
    frame #1 {
    }
  }
  n660 = while {
    tunnel: ["Bias Loop"] -> w61
    stop <- "Bias Loop" stop-if-true
    n661 = Wait (ms)(milliseconds to wait=250) -> ()  [unwired: 1 out]
    n662 = case shown="True" "Running Conditional" {
      frame #0 {
        n663 = local write "Running?"(FALSE ("Running?")) -> ()
      }
      frame #1 {
        "Running?" <- TRUE
      }
    }
  }
  n664 = local write "Compliance"(w49) -> ()
  n665 = local write "Bias Loop"(w48) -> ()
  n666 = Not(x=w61) -> (.not. x?=w60:bool)
  n667 = local write "Bias Loop"(w60) -> ()
